vi "TCP IP Command Tester.vi"() -> ()   [LabVIEW 2015]
uses:
  Controls/Control_Fornax Set Monopolar Command - Coag Mode Enum.ctl
  Controls/Control_Fornax Set Monopolar Command - Serial Number String.ctl
  Controls/Control_Fornax Set Monopolar Command - Energy Channel ID Enum.ctl
  Controls/Control_Fornax Set Monopolar Command - Cut Mode Enum.ctl
  Controls/Control_Fornax Set Monopolar Command - Cut Power Command Enum.ctl
  Controls/Control_Fornax Set Monopolar Command - Coag Power Command Enum.ctl
  Controls/Control_Fornax Source ID.ctl
  Controls/Control_Fornax Switch ID.ctl
  Controls/Control_Fornax Energy Channel ID.ctl
  Controls/Control_Fornax Switch State.ctl
  Controls/Control_Fornax Energy Mode.ctl
  Controls/Control_Fornax Parameter Value.ctl
  Controls/Control_Fornax Parameter Type.ctl
  Controls/Control_Fornax Instrument Type.ctl
  Controls/Control_Fornax Mono1 Cut Increase Power.ctl
  Controls/Control_Fornax Mono1 Cut Decrease Power.ctl
  Controls/Control_Fornax Mono1 Coag Increase Power.ctl
  Controls/Control_Fornax Mono1 Coag Decrease Power.ctl
  Controls/Control_Fornax Mono1 Cut Enum.ctl
  Controls/Control_Fornax Mono1 Coag Enum.ctl
  Controls/Control_Fornax Mono1 Cut Activate Port Bool.ctl
  Controls/Control_Fornax Mono1 Coag Activate Port Bool.ctl
  Controls/Control_Fornax Mono2 Cut Activate Port Bool.ctl
  Controls/Control_Fornax Mono2 Coag Activate Port Bool.ctl
  Controls/Control_Fornax Mono2 Cut Decrease Power.ctl
  Controls/Control_Fornax Mono2 Cut Increase Power.ctl
  Controls/Control_Fornax Mono2 Cut Enum.ctl
  Controls/Control_Fornax Mono2 Coag Decrease Power.ctl
  Controls/Control_Fornax Mono2 Coag Increase Power.ctl
  Controls/Control_Fornax Mono2 Coag Enum.ctl
  Controls/Control_Fornax Bipolar Increase Power.ctl
  Controls/Control_Fornax Bipolar Decrease Power.ctl
  Controls/Control_Fornax Bipolar Enum.ctl
  Controls/Control_Fornax Bipolar Activate Port Bool.ctl
  Controls/Control_Fornax Ligasure Activate Port Bool.ctl
  Controls/QMH Fundamentals - Message Cluster.ctl
  Controls/Control_Fornax Generator.ctl
panel:
  in  "Stop":bool
  in  "Tab Control":T1(tab)
  in  "error in (no error)":errorcluster
  out "output cluster":T2
  out "Array":T3(array[cluster])
  in  "Fornax Executable Path":path=path "C:/Program Files (x86)/Medtronic/Fornax/x86/Fornax.exe"
  in  "Action 1":bool
  in  "ExternalCommCommand":T4(ring)=enum."EXTERNAL_COMM_COMMAND_PAIR_INTEGRATION_TESTOR"
  out "Display Message":string="Wait while TCP Connection established"
  in  "Set Monopolar Command":bool
  in  "CoagMode":T5
  in  "Serial Number":T6="T5G00443DX"
  in  "EnergyChannelID":T7
  in  "CutMode":T8
  in  "CutPowerCommand":T9
  in  "CoagPowerCommand":T10
  in  "Other Read Command":bool
  out "Display Message page 2":string="Wait while TCP Connection established"
  in  "String Command":string
  in  "Send String Command":bool
  out "String":string
  in  "Numeric (0-8)":i32
  in  "Send String Array Command":bool
  out "status":bool
  out "status 2":bool
  out "value read 2":string
  in  "Slider Status Command":bool
  in  "Switch Status Command":bool
  in  "System Config":bool
  in  "External Command":bool
  in  "External Command":T4(ring)
  in  "System Config":T11(ring)
  in  "Source ID":T12
  in  "Switch ID":T13
  in  "Switch State":T14
  in  "Energy Channel ID":T15
  in  "Energy Channel ID 2":T15
  in  "Slider Position":i32
  in  "Energy Parameter Command":bool
  in  "On/Off":bool
  in  "Mode":enum16{"Cut", "Coag", "Bipolar", "Ligasure"}(ring)
  in  "Port":enum16{"Mono1", "Mono2", "Bipolar", "Ligasure"}(ring)
  in  "Energy Mode":T16
  in  "Instrument Type":T17
  in  "Parameter Type":T18
  in  "Parameter Value":T19
  in  "Energy Channel ID 3":T15
  out "value read":string
  in  "timeout ms (25000)":i32
  in  "bytes to read":i32
  in  "mode (standard)":T20(ring)
  in  "Send Read Command":bool
  out "Mono1 - Bipolar Power":string
  out "Mono2 - Cut Power":string
  out "Mono1 - Coag Power":string
  out "Mono1 - Cut Power":string
  in  "Ligasure Activate":T21
  in  "Bipolar Activate":T22
  in  "Bipolar Enum":T23
  in  "Bipolar minus":T24
  in  "Bipolar plus":T25
  in  "Mono2 Coag Enum":T26=enum."Spray"
  in  "Mono2 Coag plus":T27
  in  "Mono2 Coag minus":T28
  in  "Mono2 Cut Enum":T29
  in  "Mono2 Cut plus":T30
  in  "Mono2 Cut minus":T31
  in  "Mono2 Coag Activate":T32
  in  "Mono2 Cut Activate":T33
  in  "Mono1 Coag Activate":T34
  in  "Mono1 Cut Activate":T35
  in  "Mono1 Coag Enum":T36=enum."Spray"
  in  "Mono1 Cut Enum":T37
  in  "Mono1 Coag minus":T38
  in  "Mono1 Coag plus":T39
  in  "Mono1 Cut minus":T40
  in  "Mono1 Cut plus":T41
  out "Mono2 - Coag Power":string
  in  "Test Read":bool
  in  "Slow Read":bool
  out "value read 3":string
  out "Open Bracket Found":bool
  out "Open Bracket":string
  out "Close Bracket Found":bool
  out "Current Read":string
  in  "Timeout":dbl=5.0 format="%#_13g"
  in  "milliseconds to wait":u32=100
  out "JSON Message":string[](array[string])
  # "Mono1"
  # "Mono2"
  # "Bipolar"
  # "Ligasure"
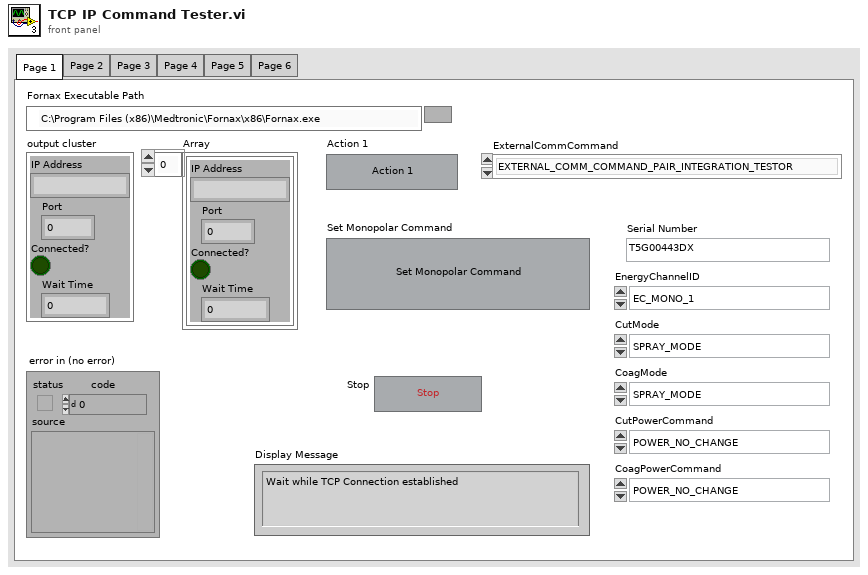
[diagram p1: front panel]
types:
  T1 = enum32{"Page 1", "Page 2", "Page 3", "Page 4", "Page 5", "Page 6"}
  T2 = cluster{"IP Address":string, "Port":u16, "Connected?":bool, "Wait Time":dbl}
  T3 = cluster{"IP Address":string, "Port":u16, "Connected?":bool, "Wait Time":dbl}[]
  T4 = enum16{"EXTERNAL_COMM_COMMAND_INVALID", "EXTERNAL_COMM_COMMAND_PAIR_VLEX", "EXTERNAL_COMM_COMMAND_PAIR_FORNAX", "EXTERNAL_COMM_COMMAND_PAIR_INTEGRATION_TESTOR", "EXTERNAL_COMM_COMMAND_ENABLE_DFA", "EXTERNAL_COMM_COMMAND_ENABLE_DFT", "EXTERNAL_COMM_COMMAND_ENABLE_VIPER", "EXTERNAL_COMM_COMMAND_AUTO_ETHERNET_ON", "EXTERNAL_COMM_COMMAND_AUTO_ETHERNET_OFF", "EXTERNAL_COMM_COMMAND_STREAM_RFDATA_ON", "EXTERNAL_COMM_COMMAND_STREAM_RFDATA_OFF", "EXTERNAL_COMM_COMMAND_STREAM_ISOFIRM_ON", "EXTERNAL_COMM_COMMAND_STREAM_ISOFIRM_OFF", "EXTERNAL_COMM_COMMAND_STREAM_RFID_ON", "EXTERNAL_COMM_COMMAND_STREAM_RFID_OFF", "EXTERNAL_COMM_COMMAND_AUTO_ETHERNET_ONCE"}
  T5 = typedef "Control_Fornax Set Monopolar Command - Coag Mode Enum.ctl" = enum16{"SPRAY_MODE", "CUT_MODE", "BLEND_MODE", "FULGERATE_MODE", "BEPOLAR_MODE", "VESSEL_SEALING_MODE", "VALLEYLAB_MODE", "BIPOLAR_RESECTION_CUT_MODE", "BIPOLAR_RESECTION_COAG_MODE", "AUTOBIPOLAR_MODE", "VIPER_HLA", "SOFT_COAG_MODE", "NUM_ENERGY_MODES"}
  T6 = typedef "Control_Fornax Set Monopolar Command - Serial Number String.ctl" = string
  T7 = typedef "Control_Fornax Set Monopolar Command - Energy Channel ID Enum.ctl" = enum16{"EC_MONO_1", "EC_BIPOLAR", "EC_MONO_2", "EC_ADVANCED", "NUM_ENERGY_CHANNELS", "EC_NOT_USED"}
  T8 = typedef "Control_Fornax Set Monopolar Command - Cut Mode Enum.ctl" = enum16{"SPRAY_MODE", "CUT_MODE", "BLEND_MODE", "FULGERATE_MODE", "BIPOLAR_MODE", "VESSEL_SEALING_MODE", "VALLEYLAB_MODE", "BIPOLAR_RESECTION_CUT_MODE", "BIPOLAR_RESECTION_COAG_MODE", "AUTOBIPOLAR_MODE", "VIPER_HLA", "SOFT_COAG_MODE", "NUM_ENERGY_MODES"}
  T9 = typedef "Control_Fornax Set Monopolar Command - Cut Power Command Enum.ctl" = enum16{"POWER_NO_CHANGE", "POWER_INCREASE", "POWER_DECREASE", "POWER_INCREASE_REPEAT", "POWER_DECREASE_REPEAT"}
  T10 = typedef "Control_Fornax Set Monopolar Command - Coag Power Command Enum.ctl" = enum16{"POWER_NO_CHANGE", "POWER_INCREASE", "POWER_DECREASE", "POWER_INCREASE_REPEAT", "POWER_DECREASE_REPEAT"}
  T11 = enum16{"SYSTEM_CONFIG_CMD_NONE", "SYSTEM_CONFIG_CMD_READ_CONFIG", "SYSTEM_CONFIG_CMD_WRITE_CONFIG", "SYSTEM_CONFIG_CMD_SW_UPDATE_ENTER", "SYSTEM_CONFIG_CMD_SW_UPDATE_START", "SYSTEM_CONFIG_CMD_SW_UPDATE_EXIT", "SYSTEM_CONFIG_CMD_UPDATE_ONE_BOARD_CHASSIS_INFO", "SYSTEM_CONFIG_CMD_UPDATE_ALL_BOARDS_CHASSIS_INFO", "SYSTEM_CONFIG_CMD_READ_ONE_BOARD_INFO", "SYSTEM_CONFIG_CMD_READ_ALL_BOARDS_INFO", "SYSTEM_CONFIG_CMD_REGISTER_BOARD", "SYSTEM_CONFIG_CMD_APPROVE_CURRENT_CONFIG", "SYSTEM_CONFIG_CMD_ROTATE_EVENT_LOGS", "SYSTEM_CONFIG_CMD_SYSTEM_RESTART", "SYSTEM_CONFIG_CMD_ROTATE_USAGE_LOGS", "SYSTEM_CONFIG_CMD_ENTER_SERVICE", "SYSTEM_CONFIG_CMD_EXIT_SERVICE", "SYSTEM_CONFIG_CMD_SW_UPDATE_CONFIRM", "SYSTEM_CONFIG_CMD_ROTATE_ALL_LOGS"}
  T12 = typedef "Control_Fornax Source ID.ctl" = enum16{"SWITCH_SOURCE_UNKNOWN  ", "SWITCH_SOURCE_HANDSWITCH  ", "SWITCH_SOURCE_FOOTSWITCH  ", "SWITCH_SOURCE_AUTO_BIPOLAR  ", "SWITCH_SOURCE_CARDIOBLATE  ", "SWITCH_SOURCE_SCREEN  ", "NUM_SWITCH_SOURCES  "}
  T13 = typedef "Control_Fornax Switch ID.ctl" = enum16{"SWITCH_ID_NONE  ", "SWITCH_ID_CUT  ", "SWITCH_ID_VMODE  ", "SWITCH_ID_COAG  ", "SWITCH_ID_LIGASURE  ", "SWITCH_ID_BIPOLAR  ", "SWITCH_ID_STAPLER_CLOSE  ", "SWITCH_ID_STAPLER_OPEN  ", "SWITCH_ID_CARDIOBLATE_BIPOLAR  ", "SWITCH_ID_CARDIOBLATE_BIPOLAR_TOUCHSCREEN  ", "SWITCH_ID_CARDIOBLATE_MONOPOLAR  ", "SWITCH_ID_CARDIOBLATE_MONOPOLAR_TOUCHSCREEN  ", "SWITCH_ID_ULTRASONIC_BTN1  ", "SWITCH_ID_ULTRASONIC_BTN2  ", "SWITCH_ID_MAX  "}
  T14 = typedef "Control_Fornax Switch State.ctl" = enum16{"SWITCH_STATE_NULL  ", "SWITCH_STATE_PRESSED  ", "SWITCH_STATE_RELEASED  ", "NUM_SWITCH_STATES  "}
  T15 = typedef "Control_Fornax Energy Channel ID.ctl" = enum16{"EC_MONO_1  ", "EC_BIPOLAR  ", "EC_MONO_2  ", "EC_ADVANCED  ", "EC_ADVANCED_ECUT  ", "EC_ADVANCED_DCUT  ", "EC_SHARED_COAG  ", "EC_INTERNAL_BIP_CAL  "}
  T16 = typedef "Control_Fornax Energy Mode.ctl" = enum16{"SPRAY_MODE", "CUT_MODE", "BLEND_MODE", "FULGERATE_MODE", "BIPOLAR_MODE", "VESSEL_SEALING_MODE", "VALLEYLAB_MODE", "BIPOLAR_RESECTION_CUT_MODE", "BIPOLAR_RESECTION_COAG_MODE", "AUTOBIPOLAR_MODE", "VIPER_HLA", "SOFT_COAG_MODE", "ECUT_MODE", "SHARED_SPRAY_MODE", "SHARED_FULGERATE_MODE", "CARDIO_MONO_MODE", "CARDIO_BIPOLAR_MODE", "BIPOLAR_LOW_MODE", "BIPOLAR_MACRO_MODE", "BIPOLAR_STANDARD_MODE", "BIPOLAR_MEDIUM_MODE", "VL_ENDOSCOPY_MODE", "NUM_ENERGY_MODES"}
  T17 = typedef "Control_Fornax Instrument Type.ctl" = enum16{"INSTRUMENT_TYPE_UNKNOWN", "INSTRUMENT_TYPE_MONOPOLAR", "INSTRUMENT_TYPE_BIPOLAR", "INSTRUMENT_TYPE_TRIVERSE", "INSTRUMENT_TYPE_LIGASURE", "INSTRUMENT_TYPE_ADVANCE_II", "INSTRUMENT_TYPE_BIPOLAR_RESECTION", "INSTRUMENT_TYPE_HOOK", "INSTRUMENT_TYPE_BIZACT", "INSTRUMENT_TYPE_CARDIOBLATE_BIP", "INSTRUMENT_TYPE_CARDIOBLATE_BIP_GEMINI_S", "INSTRUMENT_TYPE_CARDIOBLATE_MONO", "INSTRUMENT_TYPE_ULTRASONIC", "INSTRUMENT_TYPE_MONOPOLAR_GI ", "INSTRUMENT_TYPE_GOLDILOCKS "}
  T18 = typedef "Control_Fornax Parameter Type.ctl" = enum16{"POWER_PARAMETER", "CUT_MODALITY_POWER_PARAMETER", "COAG_MODALITY_POWER_PARAMETER", "VL_MODALITY_POWER_PARAMETER", "BY_MODE_POWER_PARAMETER", "VL_ENDO_CUT_MODALITY_POWER_PARAMETER", "VL_ENDO_COAG_MODALITY_POWER_PARAMETER", "VL_ENDO_COAG_ON_CUT_MODALITY_POWER_PARAMETER", "MODE_PARAMETER   (for changing Bipolar mode)", "CUT_MODALITY_MODE_PARAMETER  (for changing monopolar cut mode)", "COAG_MODALITY_MODE_PARAMETER (for changing monopolar coag mode)", "VL_ENDO_COAG_MODALITY_MODE_PARAMETER", "VL_ENDO_CUT_INTERVAL_PARAMETER", "VL_ENDO_CUT_DURATION_PARAMETER", "POWER_BAR_PARAMETER", "MAX_ACTIVATION_MSEC_TIME_PARAMETER", "AUTOBIPOLAR_DELAY_MSEC_TIME", "VL_ENDO_COAG_QUICK_ACCESS_PARAMETER"}
  T19 = typedef "Control_Fornax Parameter Value.ctl" = i32
  T20 = enum16{"Standard", "Buffered", "CRLF", "Immediate"}
  T21 = typedef "Control_Fornax Ligasure Activate Port Bool.ctl" = bool
  T22 = typedef "Control_Fornax Bipolar Activate Port Bool.ctl" = bool
  T23 = typedef "Control_Fornax Bipolar Enum.ctl" = enum16{"Standard", "Macro", "Precision"}
  T24 = typedef "Control_Fornax Bipolar Decrease Power.ctl" = bool
  T25 = typedef "Control_Fornax Bipolar Increase Power.ctl" = bool
  T26 = typedef "Control_Fornax Mono2 Coag Enum.ctl" = enum16{"Fulgerate", "Spray"}
  T27 = typedef "Control_Fornax Mono2 Coag Increase Power.ctl" = bool
  T28 = typedef "Control_Fornax Mono2 Coag Decrease Power.ctl" = bool
  T29 = typedef "Control_Fornax Mono2 Cut Enum.ctl" = enum16{"Pure", "Blend"}
  T30 = typedef "Control_Fornax Mono2 Cut Increase Power.ctl" = bool
  T31 = typedef "Control_Fornax Mono2 Cut Decrease Power.ctl" = bool
  T32 = typedef "Control_Fornax Mono2 Coag Activate Port Bool.ctl" = bool
  T33 = typedef "Control_Fornax Mono2 Cut Activate Port Bool.ctl" = bool
  T34 = typedef "Control_Fornax Mono1 Coag Activate Port Bool.ctl" = bool
  T35 = typedef "Control_Fornax Mono1 Cut Activate Port Bool.ctl" = bool
  T36 = typedef "Control_Fornax Mono1 Coag Enum.ctl" = enum16{"Fulgerate", "Spray"}
  T37 = typedef "Control_Fornax Mono1 Cut Enum.ctl" = enum16{"Pure", "Blend"}
  T38 = typedef "Control_Fornax Mono1 Coag Decrease Power.ctl" = bool
  T39 = typedef "Control_Fornax Mono1 Coag Increase Power.ctl" = bool
  T40 = typedef "Control_Fornax Mono1 Cut Decrease Power.ctl" = bool
  T41 = typedef "Control_Fornax Mono1 Cut Increase Power.ctl" = bool
  T42 = cluster{"Mono1 Cut Enum":refnum<vi>, "Mono1 - Cut Power":refnum<vi>, "Mono1 Coag Enum":refnum<vi>, "Mono1 - Coag Power":refnum<vi>, "Mono2 Cut Enum":refnum<vi>, "Mono2 - Cut Power":refnum<vi>, "Mono2 Coag Enum":refnum<vi>, "Mono2 - Coag Power":refnum<vi>, "Bipolar Enum":refnum<vi>, "Mono1 - Bipolar Power":refnum<vi>}
  T43 = typedef "QMH Fundamentals - Message Cluster.ctl" = cluster{"Message":string, "Message Data":variant}
  T44 = typedef "Control_Fornax Generator.ctl" = string
  T45 = cluster{"Port":enum16{"Mono1", "Mono2", "Bipolar", "Ligasure"}, "Mode":enum16{"Cut", "Coag", "Bipolar", "Ligasure"}, "On/Off":bool}
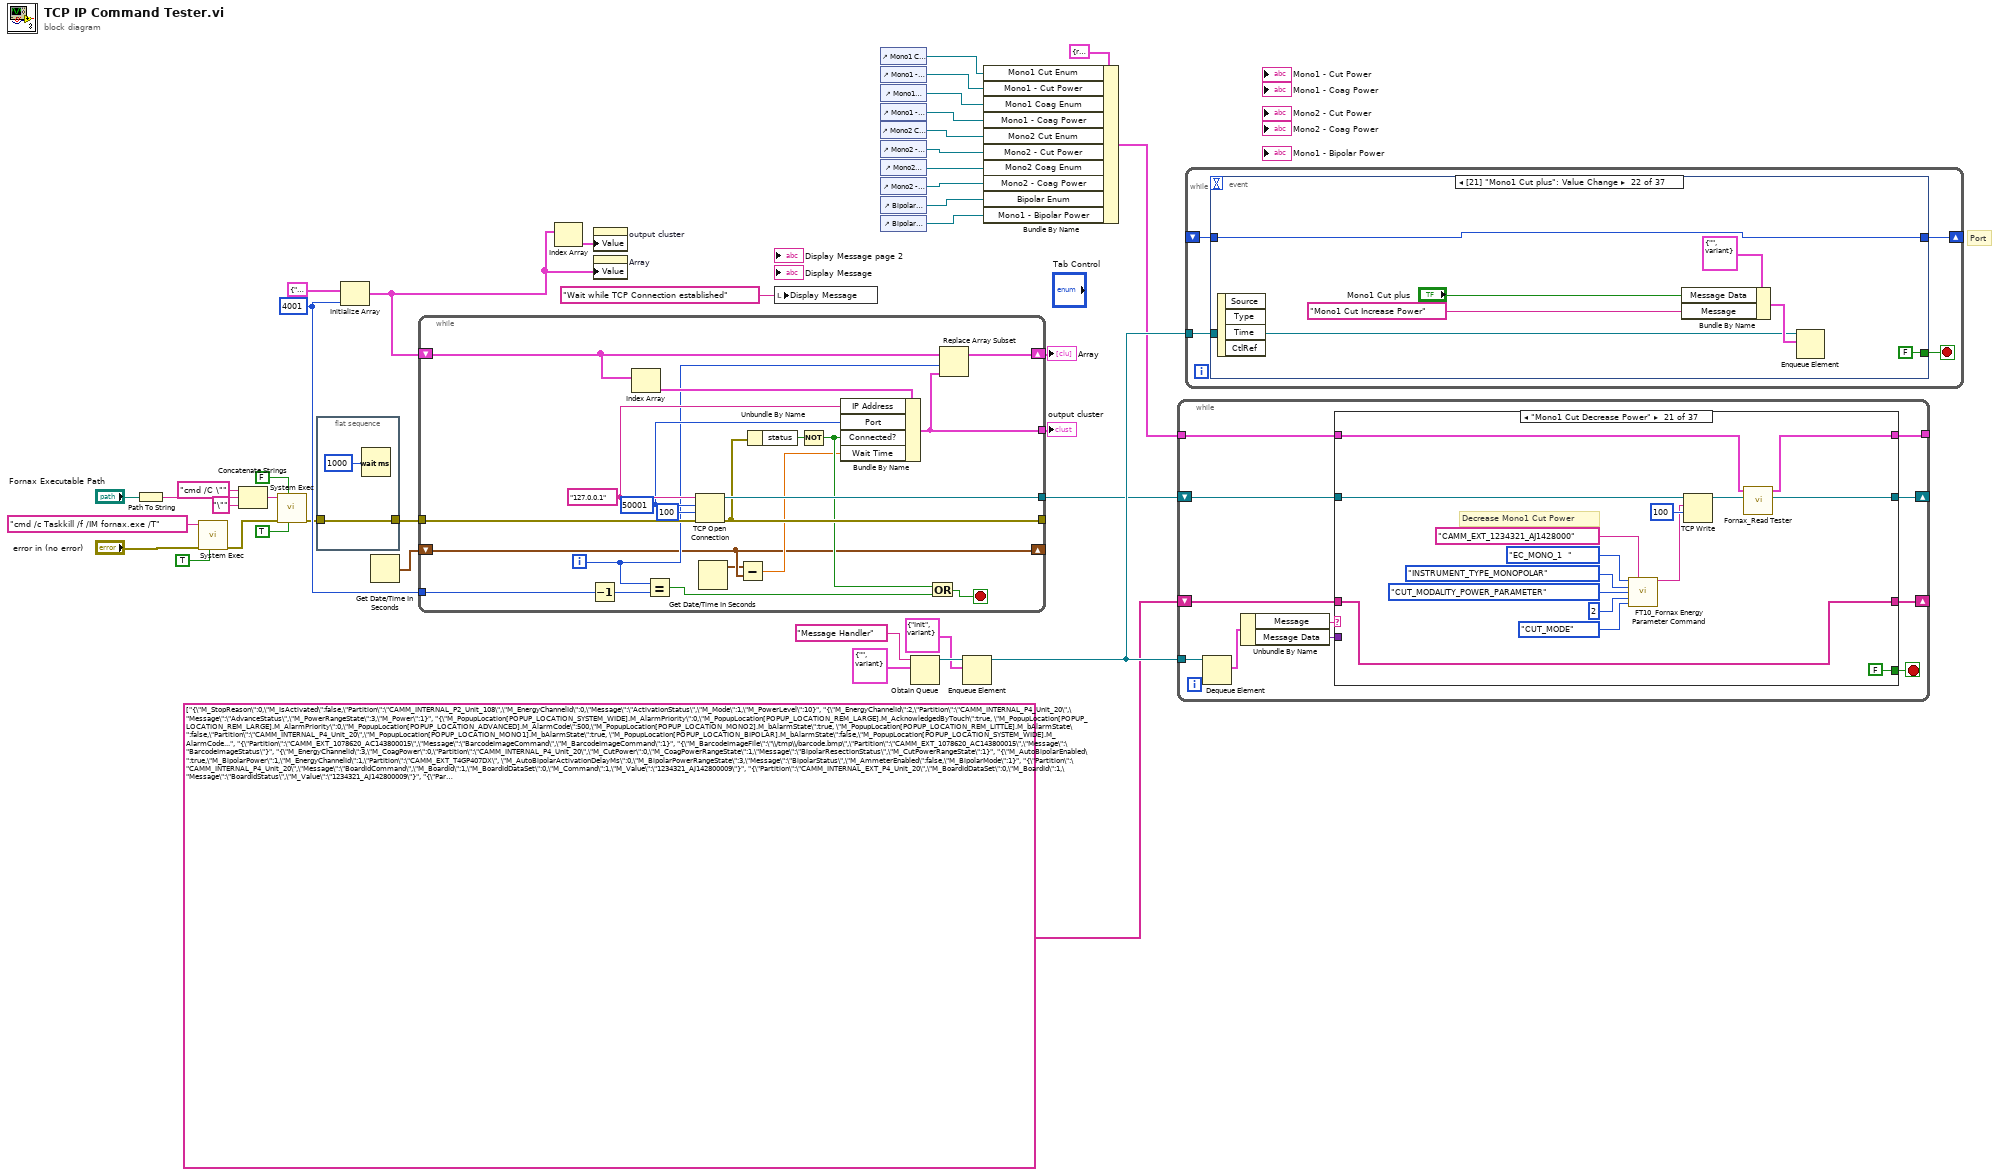
[diagram p0: block diagram]
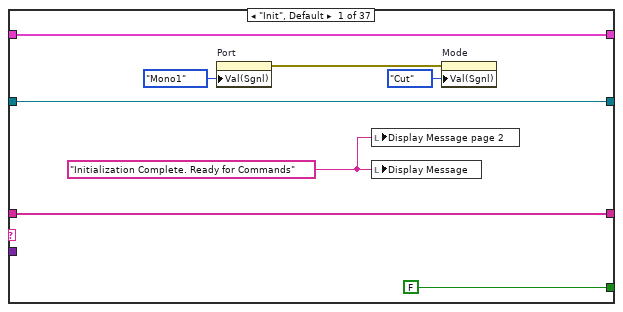
[diagram p2: hidden frame]
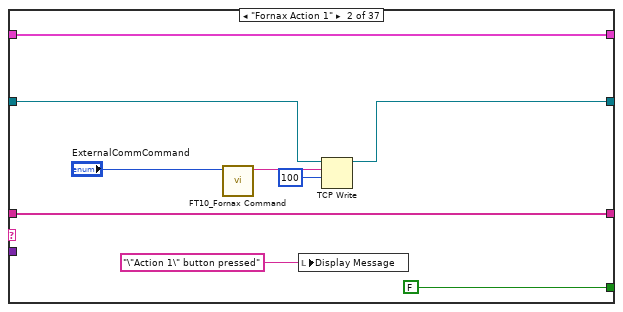
[diagram p3: hidden frame]
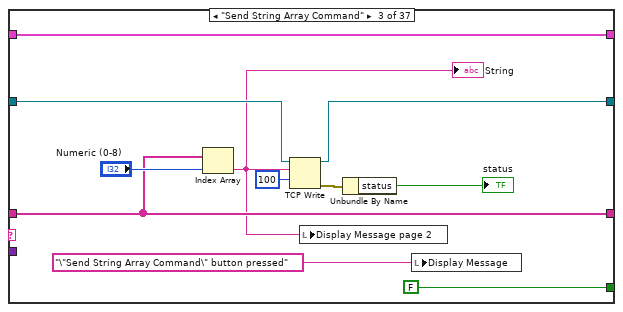
[diagram p4: hidden frame]
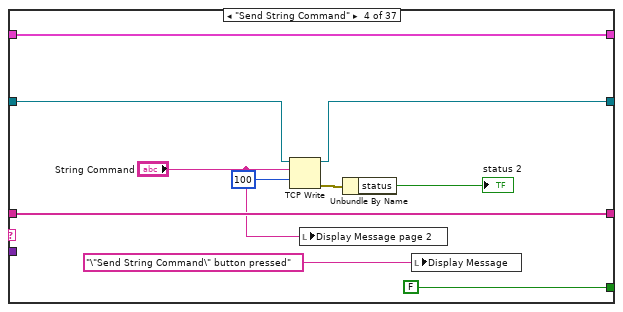
[diagram p5: hidden frame]
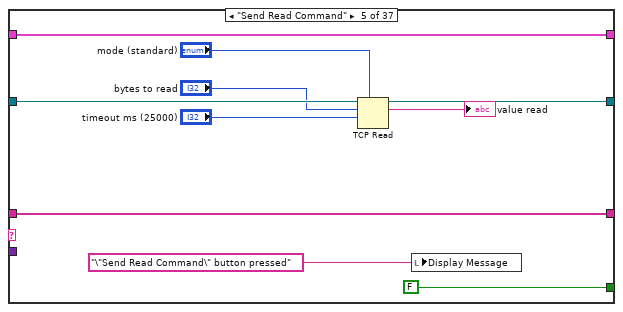
[diagram p6: hidden frame]
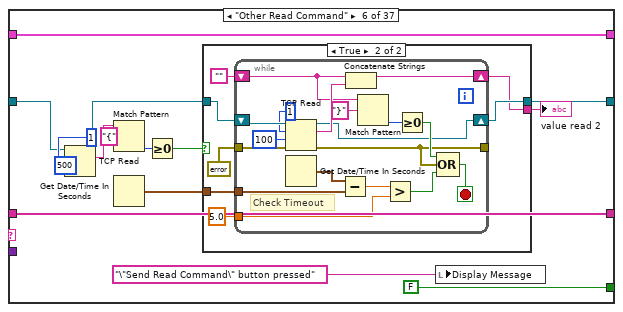
[diagram p7: hidden frame]
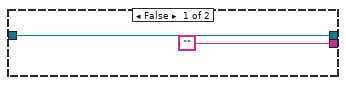
[diagram p8: hidden frame]
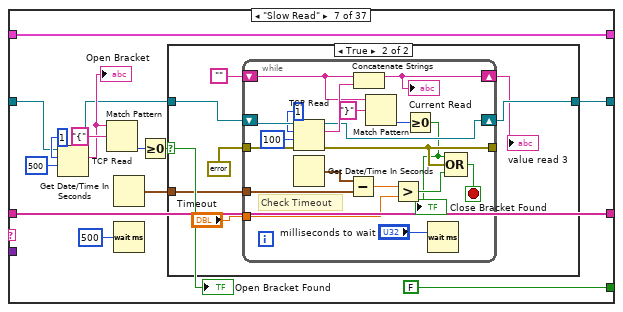
[diagram p9: hidden frame]
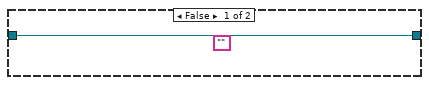
[diagram p10: hidden frame]
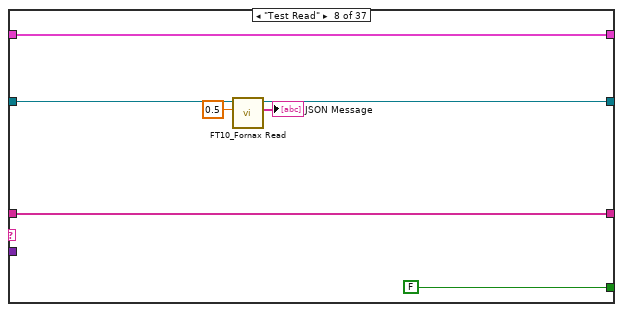
[diagram p11: hidden frame]
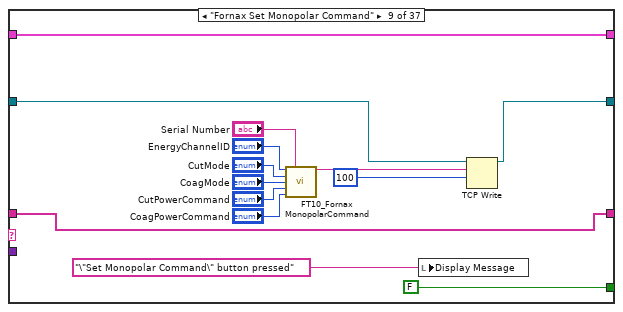
[diagram p12: hidden frame]
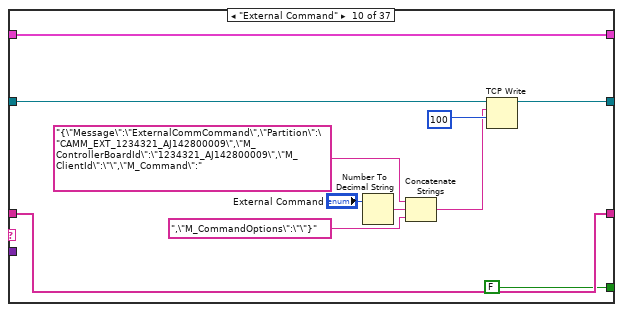
[diagram p13: hidden frame]
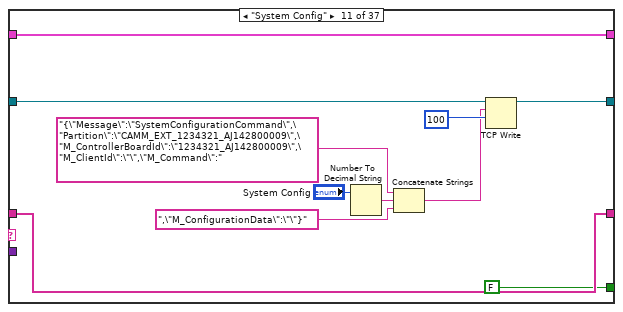
[diagram p14: hidden frame]
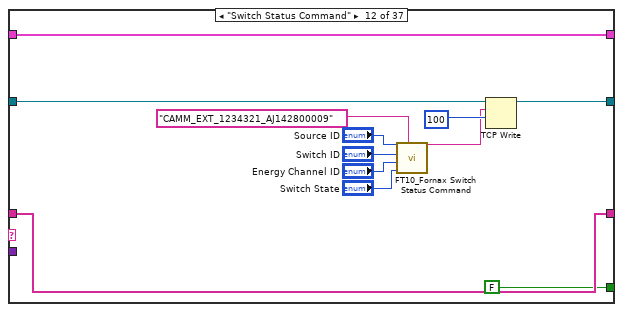
[diagram p15: hidden frame]
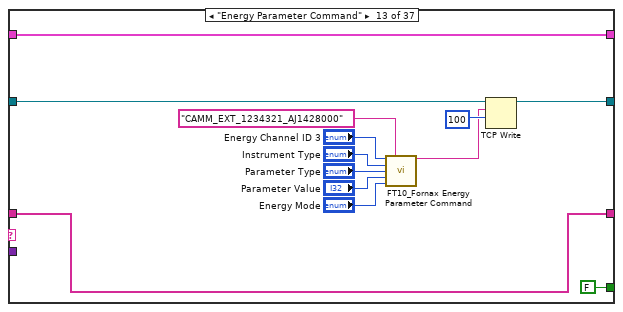
[diagram p16: hidden frame]
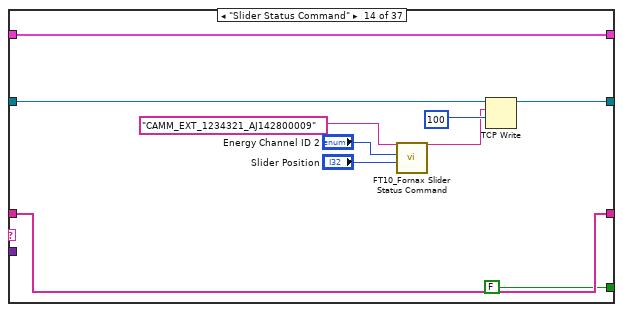
[diagram p17: hidden frame]
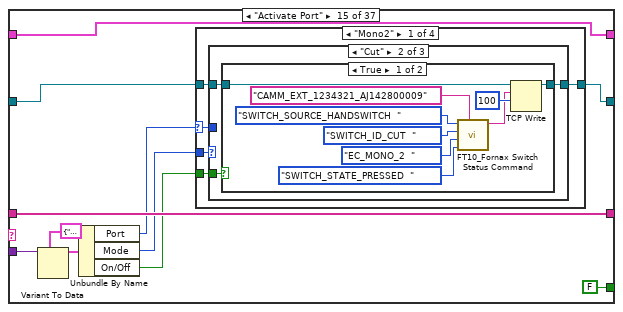
[diagram p18: hidden frame]
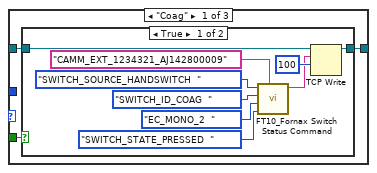
[diagram p19: hidden frame]
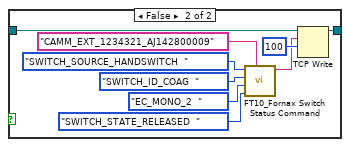
[diagram p20: hidden frame]
diagram:
  w38 = 4001 ("dimension size")
  # "Port"
  n1 = Path To String(path="Fornax Executable Path") -> (string=w27:string)
  n2 = call <vilib>:"System Exec.vi"("run minimized? (F)"=TRUE, "error in (no error)"="error in (no error)", "command line"="cmd /c Taskkill /f /IM fornax.exe /T") -> ("error out"=w33:errorcluster)  [unwired: 5 in, 3 out]
  n3 = Concatenate Strings("cmd /C \"" ("string"), w27, "\"" ("string")) -> (w29:string)
  n4 = call <vilib>:"System Exec.vi"("run minimized? (F)"=TRUE, "wait until completion? (T)"=FALSE, "error in (no error)"=w33, "command line"=w29) -> ("error out"=w13:errorcluster)  [unwired: 4 in, 3 out]
  n5 = flat-sequence {
    tunnel: [w42] -> w14
    tunnel: w13 -> [w42]
    frame #0 {
      n6 = Wait (ms)(milliseconds to wait=u32 1000) -> ()  [unwired: 1 out]
    }
  }
  n7 = Initialize Array(T2 {"IP Address"="", "Port"=0, "Connected?"=FALSE, "Wait Time"=0.0} ("Cluster"), w38) -> (w16:T3)
  n8 = Get Date/Time In Seconds() -> (seconds since 1Jan1904=w35:timestamp)
  n9 = while {
    tunnel: [w61] -> w19
    shift-right: [w60] -> w36
    shift-left: w16 -> [w59]
    tunnel: w38 -> [w50]
    tunnel: [w47] -> w37
    shift-right: [w44] -> _
    shift-left: w35 -> [w44]
    tunnel: w14 -> [w62]
    tunnel: [w55] -> _
    i -> [w46]
    stop <- w52 stop-if-true
    w56 = u16 50001 ("remote port or service name")
    w57 = "127.0.0.1" ("address")
    n10 = Decrement(x=w50) -> (x-1=w49:i32)
    n11 = Index Array(array=w59) -> (element=w58:T2)  [unwired: 1 in]
    n12 = Equal?(x=w46, y=w49) -> (x = y?=w48:bool)
    n13 = TCP Open Connection(address=w57, remote port or service name=w56, timeout ms (60000)=100, error in (no error)=w62) -> (connection ID=w61:refnum<k5>, error out=w55:errorcluster)  [unwired: 1 in]
    n14 = Get Date/Time In Seconds() -> (seconds since 1Jan1904=w43:timestamp)
    n15 = Subtract(x=w43, y=w44) -> (x-y=w45:dbl)
    n16 = Unbundle By Name(w55) -> ("status"=w54:bool)
    n17 = Not(x=w54) -> (.not. x?=w51:bool)
    n18 = Bundle By Name(cluster=w58, "IP Address"=w57, "Port"=w56, "Connected?"=w51, "Wait Time"=w45) -> (w47:T2)
    n19 = Or(x=w51, y=w48) -> (x .or. y?=w52:bool)
    n20 = Replace Array Subset(array=w59, new element=w47, index=w46) -> (w60:T3)
  }
  "output cluster" <- w37
  "Array" <- w36
  n21 = Index Array(array=w16) -> (element=w17:T2)  [unwired: 1 in]
  n22 = property on="output cluster" class="Clust (strict)"("Value"=w17) -> ()  [unwired: 2 in, 2 out]
  n23 = property on="Array" class="Arr (strict)"("Value"=w16) -> ()  [unwired: 2 in, 2 out]
  n24 = local write "Display Message"("Wait while TCP Connection established" ("Display Message")) -> ()
  n25 = control-ref of="Mono1 Cut Enum"() -> (w12:refnum<vi>)
  n26 = control-ref of="Mono1 - Cut Power"() -> (w5:refnum<vi>)
  n27 = control-ref of="Mono1 Coag Enum"() -> (w9:refnum<vi>)
  n28 = control-ref of="Mono1 - Coag Power"() -> (w4:refnum<vi>)
  n29 = control-ref of="Mono2 Cut Enum"() -> (w8:refnum<vi>)
  n30 = control-ref of="Mono2 - Cut Power"() -> (w3:refnum<vi>)
  n31 = control-ref of="Mono2 Coag Enum"() -> (w7:refnum<vi>)
  n32 = control-ref of="Mono2 - Coag Power"() -> (w2:refnum<vi>)
  n33 = control-ref of="Bipolar Enum"() -> (w6:refnum<vi>)
  n34 = control-ref of="Bipolar Power"() -> (w1:refnum<vi>)
  n35 = Obtain Queue(name (unnamed)="Message Handler", element data type=T43 {"Message"="", "Message Data"=variant} ("Message Cluster")) -> (queue out=w23:refnum<queue>)  [unwired: 3 in, 2 out]
  n36 = Enqueue Element(queue=w23, element=T43 {"Message"="Init", "Message Data"=variant}) -> (queue out=w20:refnum<queue>)  [unwired: 2 in, 2 out]
  n37 = Bundle By Name(cluster=T42 {"Mono1 Cut Enum"=refnum, "Mono1 - Cut Power"=refnum, "Mono1 Coag Enum"=refnum, "Mono1 - Coag Power"=refnum, "Mono2 Cut Enum"=refnum, "Mono2 - Cut Power"=refnum, "Mono2 Coag Enum"=refnum, "Mono2 - Coag Power"=refnum, "Bipolar Enum"=refnum, "Mono1 - Bipolar Power"=refnum}, "Mono1 Cut Enum"=w12, "Mono1 - Cut Power"=w5, "Mono1 Coag Enum"=w9, "Mono1 - Coag Power"=w4, "Mono2 Cut Enum"=w8, "Mono2 - Cut Power"=w3, "Mono2 Coag Enum"=w7, "Mono2 - Coag Power"=w2, "Bipolar Enum"=w6, "Mono1 - Bipolar Power"=w1) -> (w11:T42)
  n38 = while {
    tunnel: w20 -> [w72]
    shift-right: [w69] -> _
    shift-left: w19 -> [w68]
    shift-right: [w66] -> _
    shift-left: string[] ["{\"M_StopReason\":0,\"M_IsActivated\":false,\"Partition\":\"CAMM_INTERNAL_P2_Unit_108\",\"M_EnergyChannelId\":0,\"Message\":\"ActivationStatus\",\"M_Mode\":1,\"M_PowerLevel\":10}", "{\"M_EnergyChannelId\":2,\"Partition\":\"CAMM_INTERNAL_P4_Unit_20\",\"Message\":\"AdvanceStatus\",\"M_PowerRangeState\":3,\"M_Power\":1}", "{\"M_PopupLocation[POPUP_LOCATION_SYSTEM_WIDE].M_AlarmPriority\":0,\"M_PopupLocation[POPUP_LOCATION_REM_LARGE].M_AcknowledgedByTouch\":true, \"M_PopupLocation[POPUP_LOCATION_REM_LARGE].M_AlarmPriority\":0,\"M_PopupLocation[POPUP_LOCATION_ADVANCED].M_AlarmCode\":500,\"M_PopupLocation[POPUP_LOCATION_MONO2].M_bAlarmState\":true, \"M_PopupLocation[POPUP_LOCATION_REM_LITTLE].M_bAlarmState\":false,\"Partition\":\"CAMM_INTERNAL_P4_Unit_20\",\"M_PopupLocation[POPUP_LOCATION_MONO1].M_bAlarmState\":true, \"M_PopupLocation[POPUP_LOCATION_BIPOLAR].M_bAlarmState\":false,\"M_PopupLocation[POPUP_LOCATION_SYSTEM_WIDE].M_AlarmCode\":500,\"M_PopupLocation[POPUP_LOCATION_DEMO_MODE].M_AlarmCode\":500, \"M_PopupLocation[POPUP_LOCATION_SYSTEM_WIDE].M_AcknowledgedByTouch\":true,\"M_PopupLocation[POPUP_LOCATION_ADVANCED].M_AcknowledgedByTouch\":true, \"M_PopupLocation[POPUP_LOCATION_REM_LARGE].M_bAlarmState\":false,\"M_PopupLocation[POPUP_LOCATION_REM_LITTLE].M_AcknowledgedByTouch\":false,\"M_PopupLocation[POPUP_LOCATION_BIPOLAR].M_AlarmCode\":500, \"M_PopupLocation[POPUP_LOCATION_MONO1].M_AcknowledgedByTouch\":true,\"M_PopupLocation[POPUP_LOCATION_MONO1].M_AlarmCode\":331,\"M_PopupLocation[POPUP_LOCATION_REM_LITTLE].M_AlarmPriority\":0, \"Message\":\"AlarmPopupStatus\",\"M_PopupLocation[POPUP_LOCATION_DEMO_MODE].M_AcknowledgedByTouch\":true,\"M_PopupLocation[POPUP_LOCATION_MONO2].M_AlarmCode\":331, \"M_PopupLocation[POPUP_LOCATION_ADVANCED].M_AlarmPriority\":0,\"M_PopupLocation[POPUP_LOCATION_REM_LITTLE].M_AlarmCode\":500,\"M_PopupLocation[POPUP_LOCATION_BIPOLAR].M_AcknowledgedByTouch\":true, \"M_PopupLocation[POPUP_LOCATION_MONO1].M_AlarmPriority\":3,\"M_PopupLocation[POPUP_LOCATION_REM_LARGE].M_AlarmCode\":500,\"M_PopupLocation[POPUP_LOCATION_DEMO_MODE].M_bAlarmState\":false, \"M_PopupLocation[POPUP_LOCATION_SYSTEM_WIDE].M_bAlarmState\":false,\"M_PopupLocation[POPUP_LOCATION_MONO2].M_AcknowledgedByTouch\":true, \"M_PopupLocation[POPUP_LOCATION_BIPOLAR].M_AlarmPriority\":0,\"M_PopupLocation[POPUP_LOCATION_ADVANCED].M_bAlarmState\":false, \"M_PopupLocation[POPUP_LOCATION_DEMO_MODE].M_AlarmPriority\":0,\"M_PopupLocation[POPUP_LOCATION_MONO2].M_AlarmPriority\":3}", "{\"Partition\":\"CAMM_EXT_1078620_AC143800015\",\"Message\":\"BarcodeImageCommand\",\"M_BarcodeImageCommand\":1}", "{\"M_BarcodeImageFile\":\"\\/tmp\\/barcode.bmp\",\"Partition\":\"CAMM_EXT_1078620_AC143800015\",\"Message\":\"BarcodeImageStatus\"}", "{\"M_EnergyChannelId\":3,\"M_CoagPower\":0,\"Partition\":\"CAMM_INTERNAL_P4_Unit_20\",\"M_CutPower\":0,\"M_CoagPowerRangeState\":1,\"Message\":\"BipolarResectionStatus\",\"M_CutPowerRangeState\":1}", "{\"M_AutoBipolarEnabled\":true,\"M_BipolarPower\":1,\"M_EnergyChannelId\":1,\"Partition\":\"CAMM_EXT_T4GP407DX\", \"M_AutoBipolarActivationDelayMs\":0,\"M_BipolarPowerRangeState\":3,\"Message\":\"BipolarStatus\",\"M_AmmeterEnabled\":false,\"M_BipolarMode\":1}", "{\"Partition\":\"CAMM_INTERNAL_P4_Unit_20\",\"Message\":\"BoardIdCommand\",\"M_BoardId\":1,\"M_BoardIdDataSet\":0,\"M_Command\":1,\"M_Value\":\"1234321_AJ142800009\"}", "{\"Partition\":\"CAMM_INTERNAL_EXT_P4_Unit_20\",\"M_BoardIdDataSet\":0,\"M_BoardId\":1,\"Message\":\"BoardIdStatus\",\"M_Value\":\"1234321_AJ142800009\"}", "{\"Partition\":\"CAMM_INTERNAL_EXT_P4_Unit_20\",\"Message\":\"CardioblateBipolarStatus\",\"M_EnergyChannelId\":3,\"M_MaximumAblationTimeMS\":5,\"M_MaximumPowerLevel\":5}", "{\"Partition\":\"CAMM_INTERNAL_EXT_P4_Unit_20\",\"Message\":\"CardioblateMonopolarStatus\",\"M_CardioblateMonopolarPower\":5, \"M_CardioblateMonopolarPowerRangeState\":3,\"M_MaximumActivationTimeMS\":10,\"M_MaximumActivationTimeMSRangeState\":3}", "{\"Partition\":\"CAMM_INTERNAL_EXT_P4_Unit_20\",\"Message\":\"CardioblateSelectStatus\",\"M_SelectedEnergyChannel\":3}", "{\"Partition\":\"CAMM_EXT_1078620_AC143800015\",\"Message\":\"DftAlarmCommand\",\"M_ModuleId\":21,\"M_AlarmCode\":331, \"M_Command\":4,\"M_EnergyChannelId\":0,\"M_Message\":\"HELP\", \"M_CommandParams\":\"\",\"M_CommandOptions\":\"\"}", "{\"Partition\":\"CAMM_INTERNAL_EXT_P4_Unit_20\",\"M_AudioSequence\":1,\"Message\":\"DftAudioPlayCommand\",\"M_PlayMode\":3,\"M_Priority\":0,\"M_Volume\":50,\"M_OverrideSeqVolume\":false}", "{\"M_EnergyChannelId\":3,\"Partition\":\"CAMM_INTERNAL_EXT_P4_Unit_20\",\"Message\":\"DftInstrumentCommand\",\"M_DftInstrumentCommand\":1,\"M_IntValue\":0,\"M_FloatValue\":0.0,\"M_StringValue\":\"\"}", "{\"Partition\":\"CAMM_EXT_1078620_AC143800015\",\"Message\":\"DftLogCommand\",\"M_Command\":3,\"M_CommandOptions\":\"\"}", "{\"M_Command\":1,\"M_CalibrationType\":0,\"M_CalibrationTime\":\"\",\"M_Options\":\"\",\"M_EmA2dCalData.M_BipLowCurrentSecondary.M_Offset\":0.0,\"M_EmA2dCalData.M_BipLowCurrentPrimary.M_Gain\":1.0, \"M_EmA2dCalData.M_BipLowVoltPrimary.M_Gain\":1.0,\"Partition\":\"CAMM_INTERNAL_EXT_P4_Unit_20\",\"M_EmA2dCalData.M_BipHighVoltSecondary.M_Offset\":0.0,\"M_EmA2dCalData.M_BipLowVoltSecondary.M_Gain\":1.0, \"M_EmA2dCalData.M_BipLowVoltPrimary.M_Offset\":0.0,\"M_EmA2dCalData.M_BipHighVoltPrimary.M_Gain\":1.0,\"M_EmA2dCalData.M_MonoLowVoltPrimary.M_Offset\":0.0, \"M_EmA2dCalData.M_MonoLowVoltSecondary.M_Offset\":0.0,\"M_EmA2dCalData.M_BipHighCurrentSecondary.M_Offset\":0.0,\"M_EmA2dCalData.M_MonoLowVoltSecondary.M_Gain\":1.0, \"M_EmA2dCalData.M_BipHighCurrentPrimary.M_Gain\":1.0,\"M_EmA2dCalData.M_BipHighVoltSecondary.M_Gain\":1.0,\"M_EmA2dCalData.M_MonoHighVoltSecondary.M_Offset\":0.0, \"M_EmA2dCalData.M_BipHighCurrentPrimary.M_Offset\":0.0,\"Message\":\"EmA2dCalDataCommand\",\"M_EmA2dCalData.M_BipLowCurrentSecondary.M_Gain\":1.0, \"M_EmA2dCalData.M_BipLowCurrentPrimary.M_Offset\":0.0,\"M_EmA2dCalData.M_MonoHighVoltPrimary.M_Gain\":1.0, \"M_EmA2dCalData.M_BipHighCurrentSecondary.M_Gain\":1.0,\"M_EmA2dCalData.M_MonoHighVoltSecondary.M_Gain\":1.0, \"M_EmA2dCalData.M_BipHighVoltPrimary.M_Offset\":0.0,\"M_EmA2dCalData.M_MonoLowVoltPrimary.M_Gain\":1.0, \"M_EmA2dCalData.M_MonoHighVoltPrimary.M_Offset\":0.0,\"M_EmA2dCalData.M_BipLowVoltSecondary.M_Offset\":0.0}", "{\"M_EmA2dCalData.M_BipLowCurrentSecondary.M_Offset\":0.0,\"M_EmA2dCalData.M_BipLowCurrentPrimary.M_Gain\":1.01491,\"M_EmA2dCalData.M_BipLowVoltPrimary.M_Gain\":1.03926, \"Partition\":\"CAMM_EXT_1078620_AC143800029\",\"M_EmA2dCalData.M_BipHighVoltSecondary.M_Offset\":0.0,\"M_EmA2dCalData.M_BipLowVoltPrimary.M_Offset\":0.0, \"M_EmA2dCalData.M_BipLowVoltSecondary.M_Gain\":1.02606,\"M_EmA2dCalData.M_BipHighVoltPrimary.M_Gain\":1.03662,\"M_EmA2dCalData.M_MonoLowVoltPrimary.M_Offset\":0.0, \"M_EmA2dCalData.M_MonoLowVoltSecondary.M_Offset\":0.0,\"M_EmA2dCalData.M_BipHighCurrentSecondary.M_Offset\":0.0,\"M_EmA2dCalData.M_MonoLowVoltSecondary.M_Gain\":1.05138, \"M_EmA2dCalData.M_BipHighCurrentPrimary.M_Gain\":1.01475,\"M_EmA2dCalData.M_BipHighVoltSecondary.M_Gain\":1.02351,\"M_EmA2dCalData.M_MonoHighVoltSecondary.M_Offset\":0.0, \"M_EmA2dCalData.M_BipHighCurrentPrimary.M_Offset\":0.0,\"Message\":\"EmA2dCalDataStatus\",\"M_EmA2dCalData.M_BipLowCurrentSecondary.M_Gain\":1.0347, \"M_EmA2dCalData.M_BipLowCurrentPrimary.M_Offset\":0.0,\"M_EmA2dCalData.M_MonoHighVoltPrimary.M_Gain\":1.07264,\"M_EmA2dCalData.M_MonoHighVoltSecondary.M_Gain\":1.05568, \"M_EmA2dCalData.M_BipHighCurrentSecondary.M_Gain\":1.03478,\"M_Options\":\"\",\"M_EmA2dCalData.M_BipHighVoltPrimary.M_Offset\":0.0, \"M_CalibrationTime\":\"2014-11-18T00:26:27Z\", \"M_EmA2dCalData.M_MonoLowVoltPrimary.M_Gain\":1.06396,\"M_EmA2dCalData.M_MonoHighVoltPrimary.M_Offset\":0.0, \"M_CalibrationType\":-1,\"M_EmA2dCalData.M_BipLowVoltSecondary.M_Offset\":0.0}", "{\"Message\":\"EnergyParameterCommand\",\"Partition\":\"CAMM_EXT_1078620_AC143800015\",\"M_EnergyChannelId\":0;,\"M_InstrumentType\":1;,\"M_ParameterType\":1,\"M_ParameterValue\":3,\"M_EnergyMode\":-1}", "{\"Message\":\"ExternalCommCommand\",\"Partition\":\"CAMM_EXT_1078620_AC143800015\",\"M_ControllerBoardId\":\"1078620_AC143800015\",\"M_ClientId\":\"\",\"M_Command\":5,\"M_CommandOptions\":\"\"}"] ("String") -> [w65]
    tunnel: w11 -> [w63]
    tunnel: [w64] -> _
    stop <- w67 stop-if-true
    n39 = Dequeue Element(queue=w72) -> (element=w73:T43)  [unwired: 2 in, 3 out]
    n40 = Unbundle By Name(w73) -> ("Message"=w71:string, "Message Data"=w70:variant)
    n41 = case shown="\"Mono1 Cut Decrease Power\"" w71 {
      tunnel: w70 -> [_ _ _ _ _ _ _ _ _ _ _ _ _ _ w289 w455 _ _ w495 w505 _ _ w545 w555 _ _ w595 w605 _ _ w645 w655 _ _ w695 w705 _]
      tunnel: [w81 w86 w100 w110 w117 w134 w176 w207 w223 w235 w246 w258 w271 w281 w292 w452 w458 w474 w488 w501 w508 w523 w538 w550 w558 w573 w588 w599 w608 w623 w638 w649 w658 w673 w688 w700 w708] -> w69
      tunnel: w68 -> [w81 w87 w101 w111 w121 w126 w169 w208 w224 w236 w247 w259 w272 w282 w293 w453 w463 w484 w496 w502 w519 w534 w546 w551 w569 w584 w596 w600 w619 w634 w646 w651 w669 w684 w696 w702 w708]
      tunnel: [FALSE FALSE FALSE FALSE FALSE FALSE FALSE FALSE FALSE FALSE FALSE FALSE FALSE FALSE FALSE FALSE FALSE FALSE FALSE FALSE FALSE FALSE FALSE FALSE FALSE FALSE FALSE FALSE FALSE FALSE FALSE FALSE FALSE FALSE FALSE FALSE TRUE] -> w67
      tunnel: [w79 w83 w96 w107 w118 w123 w167 w209 w213 w233 w244 w256 w269 w279 w291 w451 w461 w476 w492 w504 w518 w533 w544 w554 w568 w583 w594 w604 w618 w633 w644 w654 w668 w683 w694 w704 w707] -> w66
      tunnel: w65 -> [w79 w83 w96 w107 w118 w123 w167 w209 w213 w233 w244 w256 w269 w279 w291 w451 w461 w476 w492 w504 w518 w533 w544 w554 w568 w583 w594 w604 w618 w633 w644 w654 w668 w683 w694 w704 w707]
      tunnel: [w74 w82 w91 w102 w112 w132 w175 w210 w212 w226 w237 w248 w260 w273 w283 w448 w456 w471 w486 w498 w506 w521 w536 w548 w556 w571 w586 w598 w606 w621 w636 w648 w656 w671 w686 w698 w706] -> w64
      tunnel: w63 -> [w74 w82 w91 w102 w112 w132 w175 w210 w212 w226 w237 w248 w260 w273 w283 w448 w457 w472 w487 w498 w507 w522 w537 w548 w557 w572 w587 w598 w607 w622 w637 w648 w657 w672 w687 w698 w706]
      frame "Init", Default {
        w78 = "Initialization Complete. Ready for Commands" ("Display Message")
        n42 = property on="Port" class="Enum (strict)"("Val(Sgnl)"=enum16{"Mono1", "Mono2", "Bipolar", "Ligasure"}."Mono1" ("Value (Signaling)")) -> (error out=w75:errorcluster)  [unwired: 2 in, 1 out]
        n43 = local write "Display Message page 2"(w78) -> ()
        n44 = local write "Display Message"(w78) -> ()
        n45 = property on="Mode" class="Enum (strict)"(error in=w75, "Val(Sgnl)"=enum16{"Cut", "Coag", "Bipolar", "Ligasure"}."Cut" ("Value (Signaling)")) -> ()  [unwired: 1 in, 2 out]
      }
      frame "Fornax Action 1" {
        n46 = call "FT10_Fornax Command.vi"("ExternalCommCommand"="ExternalCommCommand") -> ("JSON Message"=w89:string)  [unwired: 10 in]
        n47 = local write "Display Message"("\"Action 1\" button pressed" ("Display Message")) -> ()
        n48 = TCP Write(connection ID=w87, data in=w89, 9:100 ("timeout ms (25000)")) -> (connection ID out=w86:refnum<k5>)  [unwired: 1 in, 2 out]
      }
      frame "Send String Array Command" {
        n49 = Index Array(array=w96, index="Numeric (0-8)") -> (element=w92:string)
        "String" <- w92
        n50 = TCP Write(connection ID=w101, data in=w92, 9:100 ("timeout ms (25000)")) -> (connection ID out=w100:refnum<k5>, error out=w94:errorcluster)  [unwired: 1 in, 1 out]
        n51 = local write "Display Message page 2"(w92) -> ()
        n52 = Unbundle By Name(w94) -> ("status"=→"status":bool)
        n53 = local write "Display Message"("\"Send String Array Command\" button pressed" ("Display Message")) -> ()
      }
      frame "Send String Command" {
        n54 = TCP Write(connection ID=w111, data in="String Command", 9:100 ("timeout ms (25000)")) -> (connection ID out=w110:refnum<k5>, error out=w105:errorcluster)  [unwired: 1 in, 1 out]
        n55 = local write "Display Message page 2"("String Command") -> ()
        n56 = Unbundle By Name(w105) -> ("status"=→"status 2":bool)
        n57 = local write "Display Message"("\"Send String Command\" button pressed" ("Display Message")) -> ()
      }
      frame "Send Read Command" {
        n58 = TCP Read(connection ID=w121, bytes to read="bytes to read", 7:"mode (standard)", 9:"timeout ms (25000)") -> (connection ID out=w117:refnum<k5>, data out=→"value read":string)  [unwired: 1 in, 1 out]
        n59 = local write "Display Message"("\"Send Read Command\" button pressed" ("Display Message")) -> ()
      }
      frame "Other Read Command" {
        n60 = TCP Read(connection ID=w126, bytes to read=1, 9:500) -> (connection ID out=w125:refnum<k5>, data out=w127:string)  [unwired: 2 in, 1 out]
        n61 = Match Pattern(string=w127, regular expression="{") -> (offset past match=w128:i32)  [unwired: 1 in, 3 out]
        n62 = Get Date/Time In Seconds() -> (seconds since 1Jan1904=w122:timestamp)
        n63 = Greater Or Equal To 0?(x=w128) -> (x >= 0?=w124:bool)
        n64 = case shown="True" w124 {
          tunnel: [w138 w144] -> w134
          tunnel: ["" w143] -> w133
          tunnel: w125 -> [w138 w145]
          tunnel: w122 -> [_ w139]
          frame False {
          }
          frame True {
            n65 = while {
              tunnel: errorcluster {"status"=FALSE, "code"=0, "source"=""} ("error out") -> [w163]
              tunnel: [w149] -> _
              tunnel: w139 -> [w152]
              tunnel: 5.0 ("Timeout") -> [w159]
              shift-right: [w155] -> w143
              shift-left: "" -> [w148]
              shift-right: [w146] -> w144
              shift-left: w145 -> [w162]
              stop <- w157 stop-if-true
              # "Check Timeout"
              n66 = TCP Read(connection ID=w162, bytes to read=1, error in (no error)=w163, 9:100 ("timeout ms (25000)")) -> (connection ID out=w146:refnum<k5>, data out=w156:string, error out=w149:errorcluster)  [unwired: 1 in]
              n67 = Get Date/Time In Seconds() -> (seconds since 1Jan1904=w151:timestamp)
              n68 = Subtract(x=w151, y=w152) -> (x-y=w160:dbl)
              n69 = Concatenate Strings(w148, w156) -> (w155:string)
              n70 = Match Pattern(string=w148, regular expression="}") -> (offset past match=w161:i32)  [unwired: 1 in, 3 out]
              n71 = Greater?(x=w160, y=w159) -> (0:w158:bool)
              n72 = Greater Or Equal To 0?(x=w161) -> (x >= 0?=w150:bool)
              n73 = Compound Arithmetic op=OR(w150, w149, w158) -> (w157:bool)
            }
          }
        }
        "value read 2" <- w133
        n74 = local write "Display Message"("\"Send Read Command\" button pressed" ("Display Message")) -> ()
      }
      frame "Slow Read" {
        n75 = TCP Read(connection ID=w169, bytes to read=1, 9:500) -> (connection ID out=w168:refnum<k5>, data out=w170:string)  [unwired: 2 in, 1 out]
        "Open Bracket" <- w170
        n76 = Match Pattern(string=w170, regular expression="{") -> (offset past match=w171:i32)  [unwired: 1 in, 3 out]
        n77 = Get Date/Time In Seconds() -> (seconds since 1Jan1904=w166:timestamp)
        n78 = Wait (ms)(milliseconds to wait=u32 500) -> ()  [unwired: 1 out]
        n79 = Greater Or Equal To 0?(x=w171) -> (x >= 0?=w164:bool)
        "Open Bracket Found" <- w164
        n80 = case shown="True" w164 {
          tunnel: [w178 w184] -> w176
          tunnel: w168 -> [w178 w185]
          tunnel: w166 -> [_ w181]
          frame False {
            (unwired) ""
          }
          frame True {
            n81 = while {
              tunnel: errorcluster {"status"=FALSE, "code"=0, "source"=""} ("error out") -> [w204]
              tunnel: [w192] -> _
              tunnel: w181 -> [w194]
              tunnel: "Timeout" -> [w200]
              shift-right: [w186] -> w180
              shift-left: "" -> [w191]
              shift-right: [w189] -> w184
              shift-left: w185 -> [w203]
              stop <- w198 stop-if-true
              # "Check Timeout"
              n82 = TCP Read(connection ID=w203, bytes to read=1, error in (no error)=w204, 9:100 ("timeout ms (25000)")) -> (connection ID out=w189:refnum<k5>, data out=w197:string, error out=w192:errorcluster)  [unwired: 1 in]
              n83 = Get Date/Time In Seconds() -> (seconds since 1Jan1904=w193:timestamp)
              n84 = Subtract(x=w193, y=w194) -> (x-y=w201:dbl)
              n85 = Concatenate Strings(w191, w197) -> (w186:string)
              "Current Read" <- w186
              n86 = Match Pattern(string=w191, regular expression="}") -> (offset past match=w202:i32)  [unwired: 1 in, 3 out]
              n87 = Greater?(x=w201, y=w200) -> (0:w199:bool)
              n88 = Greater Or Equal To 0?(x=w202) -> (x >= 0?=w187:bool)
              "Close Bracket Found" <- w187
              n89 = Wait (ms)(milliseconds to wait="milliseconds to wait") -> ()  [unwired: 1 out]
              n90 = Compound Arithmetic op=OR(w187, w192, w199) -> (w198:bool)
            }
            "value read 3" <- w180
          }
        }
      }
      frame "Test Read" {
        n91 = call "FT10_Fornax Read.vi"("Timeout"=0.5, "TCP Network Connection in"=w208) -> ("JSON Message"=→"JSON Message":string[], "TCP Network Connection out"=w207:refnum<k5>)  [unwired: 7 in, 1 out]
      }
      frame "Fornax Set Monopolar Command" {
        n92 = call "FT10_Fornax MonopolarCommand.vi"("EnergyChannelID"="EnergyChannelID", "Serial Number"="Serial Number", "CutMode"="CutMode", "CoagMode"="CoagMode", "CutPowerCommand"="CutPowerCommand", "CoagPowerCommand"="CoagPowerCommand") -> ("JSON Command"=w220:string)  [unwired: 9 in]
        n93 = local write "Display Message"("\"Set Monopolar Command\" button pressed" ("Display Message")) -> ()
        n94 = TCP Write(connection ID=w224, data in=w220, 9:100 ("timeout ms (25000)")) -> (connection ID out=w223:refnum<k5>)  [unwired: 1 in, 2 out]
      }
      frame "External Command" {
        n95 = Number To Decimal String(number="External Command") -> (decimal integer string=w231:string)  [unwired: 1 in]
        n96 = Concatenate Strings("{\"Message\":\"ExternalCommCommand\",\"Partition\":\"CAMM_EXT_1234321_AJ142800009\",\"M_ControllerBoardId\":\"1234321_AJ142800009\",\"M_ClientId\":\"\",\"M_Command\":", w231, ",\"M_CommandOptions\":\"\"}") -> (w228:string)
        n97 = TCP Write(connection ID=w236, data in=w228, 9:100 ("timeout ms (25000)")) -> (connection ID out=w235:refnum<k5>)  [unwired: 1 in, 2 out]
      }
      frame "System Config" {
        n98 = Number To Decimal String(number="System Config") -> (decimal integer string=w242:string)  [unwired: 1 in]
        n99 = Concatenate Strings("{\"Message\":\"SystemConfigurationCommand\",\"Partition\":\"CAMM_EXT_1234321_AJ142800009\",\"M_ControllerBoardId\":\"1234321_AJ142800009\",\"M_ClientId\":\"\",\"M_Command\":", w242, ",\"M_ConfigurationData\":\"\"}") -> (w239:string)
        n100 = TCP Write(connection ID=w247, data in=w239, 9:100 ("timeout ms (25000)")) -> (connection ID out=w246:refnum<k5>)  [unwired: 1 in, 2 out]
      }
      frame "Switch Status Command" {
        n101 = call "FT10_Fornax Switch Status Command.vi"("Generator"=T44 "CAMM_EXT_1234321_AJ142800009", "Switch State"="Switch State", "Energy Channel ID"="Energy Channel ID", "Switch ID"="Switch ID", "Source ID"="Source ID") -> ("JSON Command"=w249:string)  [unwired: 6 in]
        n102 = TCP Write(connection ID=w259, data in=w249, 9:100 ("timeout ms (25000)")) -> (connection ID out=w258:refnum<k5>)  [unwired: 1 in, 2 out]
      }
      frame "Energy Parameter Command" {
        n103 = call "FT10_Fornax Energy Parameter Command.vi"("Energy Channel ID"="Energy Channel ID 3", "Generator"=T44 "CAMM_EXT_1234321_AJ1428000", "Instrument Type"="Instrument Type", "Parameter Type"="Parameter Type", "Parameter Value"="Parameter Value", "Energy Mode"="Energy Mode") -> ("JSON Command"=w261:string)  [unwired: 9 in]
        n104 = TCP Write(connection ID=w272, data in=w261, 9:100 ("timeout ms (25000)")) -> (connection ID out=w271:refnum<k5>)  [unwired: 1 in, 2 out]
      }
      frame "Slider Status Command" {
        n105 = call "FT10_Fornax Slider Status Command.vi"("Slider Position"="Slider Position", "Energy Channel ID"="Energy Channel ID 2", "Generator"=T44 "CAMM_EXT_1234321_AJ142800009") -> ("JSON Command"=w277:string)  [unwired: 8 in]
        n106 = TCP Write(connection ID=w282, data in=w277, 9:100 ("timeout ms (25000)")) -> (connection ID out=w281:refnum<k5>)  [unwired: 1 in, 2 out]
      }
      frame "Activate Port" {
        n107 = Variant To Data(type=T45 {"Port"=enum."Bipolar", "Mode"=enum."Bipolar", "On/Off"=FALSE}, Variant=w289) -> (data=w287:T45)  [unwired: 1 in, 1 out]
        n108 = Unbundle By Name(w287) -> ("Port"=w286:enum16{"Mono1", "Mono2", "Bipolar", "Ligasure"}, "Mode"=w285:enum16{"Cut", "Coag", "Bipolar", "Ligasure"}, "On/Off"=w284:bool)
        n109 = case shown="\"Mono2\"" w286 {
          selector: w286 -> [w296 w345 w394 w422]
          tunnel: w293 -> [w298 w347 w396 w424]
          tunnel: [w297 w346 w395 w423] -> w292
          tunnel: w285 -> [w295 w344 w393 w421]
          tunnel: w284 -> [w294 w343 w392 w420]
          frame "Mono2" {
            n110 = case shown="\"Cut\"" w295 {
              tunnel: w298 -> [w301 w322 w342]
              tunnel: [w300 w321 w342] -> w297
              tunnel: w296 -> [_ _ _]
              tunnel: w294 -> [w299 w320 _]
              frame "Coag" {
                n111 = case shown="True" w299 {
                  tunnel: w301 -> [w310 w319]
                  tunnel: [w309 w318] -> w300
                  frame True {
                    n112 = call "FT10_Fornax Switch Status Command.vi"("Generator"=T44 "CAMM_EXT_1234321_AJ142800009", "Switch State"=Control_Fornax_Switch_State."SWITCH_STATE_PRESSED  ", "Energy Channel ID"=Control_Fornax_Energy_Channel_ID."EC_MONO_2  ", "Switch ID"=Control_Fornax_Switch_ID."SWITCH_ID_COAG  ", "Source ID"=Control_Fornax_Source_ID."SWITCH_SOURCE_HANDSWITCH  ") -> ("JSON Command"=w302:string)  [unwired: 6 in]
                    n113 = TCP Write(connection ID=w310, data in=w302, 9:100 ("timeout ms (25000)")) -> (connection ID out=w309:refnum<k5>)  [unwired: 1 in, 2 out]
                  }
                  frame False {
                    n114 = call "FT10_Fornax Switch Status Command.vi"("Generator"=T44 "CAMM_EXT_1234321_AJ142800009", "Switch State"=Control_Fornax_Switch_State."SWITCH_STATE_RELEASED  ", "Energy Channel ID"=Control_Fornax_Energy_Channel_ID."EC_MONO_2  ", "Switch ID"=Control_Fornax_Switch_ID."SWITCH_ID_COAG  ", "Source ID"=Control_Fornax_Source_ID."SWITCH_SOURCE_HANDSWITCH  ") -> ("JSON Command"=w311:string)  [unwired: 6 in]
                    n115 = TCP Write(connection ID=w319, data in=w311, 9:100 ("timeout ms (25000)")) -> (connection ID out=w318:refnum<k5>)  [unwired: 1 in, 2 out]
                  }
                }
              }
              frame "Cut" {
                n116 = case shown="True" w320 {
                  tunnel: w322 -> [w331 w340]
                  tunnel: [w330 w339] -> w321
                  frame True {
                    n117 = call "FT10_Fornax Switch Status Command.vi"("Generator"=T44 "CAMM_EXT_1234321_AJ142800009", "Switch State"=Control_Fornax_Switch_State."SWITCH_STATE_PRESSED  ", "Energy Channel ID"=Control_Fornax_Energy_Channel_ID."EC_MONO_2  ", "Switch ID"=Control_Fornax_Switch_ID."SWITCH_ID_CUT  ", "Source ID"=Control_Fornax_Source_ID."SWITCH_SOURCE_HANDSWITCH  ") -> ("JSON Command"=w323:string)  [unwired: 6 in]
                    n118 = TCP Write(connection ID=w331, data in=w323, 9:100 ("timeout ms (25000)")) -> (connection ID out=w330:refnum<k5>)  [unwired: 1 in, 2 out]
                  }
                  frame False {
                    n119 = call "FT10_Fornax Switch Status Command.vi"("Generator"=T44 "CAMM_EXT_1234321_AJ142800009", "Switch State"=Control_Fornax_Switch_State."SWITCH_STATE_RELEASED  ", "Energy Channel ID"=Control_Fornax_Energy_Channel_ID."EC_MONO_2  ", "Switch ID"=Control_Fornax_Switch_ID."SWITCH_ID_CUT  ", "Source ID"=Control_Fornax_Source_ID."SWITCH_SOURCE_HANDSWITCH  ") -> ("JSON Command"=w332:string)  [unwired: 6 in]
                    n120 = TCP Write(connection ID=w340, data in=w332, 9:100 ("timeout ms (25000)")) -> (connection ID out=w339:refnum<k5>)  [unwired: 1 in, 2 out]
                  }
                }
              }
              frame Default {
                n121 = One Button Dialog(message="This mode is not allowed for this port") -> ()  [unwired: 1 in, 1 out]
              }
            }
          }
          frame "Mono1" {
            n122 = case shown="\"Coag\"" w344 {
              tunnel: w347 -> [w350 w371 w391]
              tunnel: [w349 w370 w391] -> w346
              tunnel: w345 -> [_ _ _]
              tunnel: w343 -> [w348 w369 _]
              frame "Coag" {
                n123 = case shown="False" w348 {
                  tunnel: w350 -> [w359 w368]
                  tunnel: [w358 w367] -> w349
                  frame True {
                    n124 = call "FT10_Fornax Switch Status Command.vi"("Generator"=T44 "CAMM_EXT_1234321_AJ142800009", "Switch State"=Control_Fornax_Switch_State."SWITCH_STATE_PRESSED  ", "Energy Channel ID"=Control_Fornax_Energy_Channel_ID."EC_MONO_1  ", "Switch ID"=Control_Fornax_Switch_ID."SWITCH_ID_COAG  ", "Source ID"=Control_Fornax_Source_ID."SWITCH_SOURCE_HANDSWITCH  ") -> ("JSON Command"=w351:string)  [unwired: 6 in]
                    n125 = TCP Write(connection ID=w359, data in=w351, 9:100 ("timeout ms (25000)")) -> (connection ID out=w358:refnum<k5>)  [unwired: 1 in, 2 out]
                  }
                  frame False {
                    n126 = call "FT10_Fornax Switch Status Command.vi"("Generator"=T44 "CAMM_EXT_1234321_AJ142800009", "Switch State"=Control_Fornax_Switch_State."SWITCH_STATE_RELEASED  ", "Energy Channel ID"=Control_Fornax_Energy_Channel_ID."EC_MONO_1  ", "Switch ID"=Control_Fornax_Switch_ID."SWITCH_ID_COAG  ", "Source ID"=Control_Fornax_Source_ID."SWITCH_SOURCE_HANDSWITCH  ") -> ("JSON Command"=w360:string)  [unwired: 6 in]
                    n127 = TCP Write(connection ID=w368, data in=w360, 9:100 ("timeout ms (25000)")) -> (connection ID out=w367:refnum<k5>)  [unwired: 1 in, 2 out]
                  }
                }
              }
              frame "Cut" {
                n128 = case shown="True" w369 {
                  tunnel: w371 -> [w380 w389]
                  tunnel: [w379 w388] -> w370
                  frame True {
                    n129 = call "FT10_Fornax Switch Status Command.vi"("Generator"=T44 "CAMM_EXT_1234321_AJ142800009", "Switch State"=Control_Fornax_Switch_State."SWITCH_STATE_PRESSED  ", "Energy Channel ID"=Control_Fornax_Energy_Channel_ID."EC_MONO_1  ", "Switch ID"=Control_Fornax_Switch_ID."SWITCH_ID_CUT  ", "Source ID"=Control_Fornax_Source_ID."SWITCH_SOURCE_HANDSWITCH  ") -> ("JSON Command"=w372:string)  [unwired: 6 in]
                    n130 = TCP Write(connection ID=w380, data in=w372, 9:100 ("timeout ms (25000)")) -> (connection ID out=w379:refnum<k5>)  [unwired: 1 in, 2 out]
                  }
                  frame False {
                    n131 = call "FT10_Fornax Switch Status Command.vi"("Generator"=T44 "CAMM_EXT_1234321_AJ142800009", "Switch State"=Control_Fornax_Switch_State."SWITCH_STATE_RELEASED  ", "Energy Channel ID"=Control_Fornax_Energy_Channel_ID."EC_MONO_1  ", "Switch ID"=Control_Fornax_Switch_ID."SWITCH_ID_CUT  ", "Source ID"=Control_Fornax_Source_ID."SWITCH_SOURCE_HANDSWITCH  ") -> ("JSON Command"=w381:string)  [unwired: 6 in]
                    n132 = TCP Write(connection ID=w389, data in=w381, 9:100 ("timeout ms (25000)")) -> (connection ID out=w388:refnum<k5>)  [unwired: 1 in, 2 out]
                  }
                }
              }
              frame Default {
                n133 = One Button Dialog(message="This mode is not allowed for this port") -> ()  [unwired: 1 in, 1 out]
              }
            }
          }
          frame "Bipolar" {
            n134 = case shown="\"Bipolar\"" w393 {
              tunnel: w396 -> [w399 w419]
              tunnel: [w398 w419] -> w395
              tunnel: w394 -> [_ _]
              tunnel: w392 -> [w397 _]
              frame "Bipolar" {
                n135 = case shown="False" w397 {
                  tunnel: w399 -> [w408 w417]
                  tunnel: [w407 w416] -> w398
                  frame True {
                    n136 = call "FT10_Fornax Switch Status Command.vi"("Generator"=T44 "CAMM_EXT_1234321_AJ142800009", "Switch State"=Control_Fornax_Switch_State."SWITCH_STATE_PRESSED  ", "Energy Channel ID"=Control_Fornax_Energy_Channel_ID."EC_BIPOLAR  ", "Switch ID"=Control_Fornax_Switch_ID."SWITCH_ID_BIPOLAR  ", "Source ID"=Control_Fornax_Source_ID."SWITCH_SOURCE_HANDSWITCH  ") -> ("JSON Command"=w400:string)  [unwired: 6 in]
                    n137 = TCP Write(connection ID=w408, data in=w400, 9:100 ("timeout ms (25000)")) -> (connection ID out=w407:refnum<k5>)  [unwired: 1 in, 2 out]
                  }
                  frame False {
                    n138 = call "FT10_Fornax Switch Status Command.vi"("Generator"=T44 "CAMM_EXT_1234321_AJ142800009", "Switch State"=Control_Fornax_Switch_State."SWITCH_STATE_RELEASED  ", "Energy Channel ID"=Control_Fornax_Energy_Channel_ID."EC_BIPOLAR  ", "Switch ID"=Control_Fornax_Switch_ID."SWITCH_ID_BIPOLAR  ", "Source ID"=Control_Fornax_Source_ID."SWITCH_SOURCE_HANDSWITCH  ") -> ("JSON Command"=w409:string)  [unwired: 6 in]
                    n139 = TCP Write(connection ID=w417, data in=w409, 9:100 ("timeout ms (25000)")) -> (connection ID out=w416:refnum<k5>)  [unwired: 1 in, 2 out]
                  }
                }
              }
              frame Default {
                n140 = One Button Dialog(message="This mode is not allowed for this port") -> ()  [unwired: 1 in, 1 out]
              }
            }
          }
          frame "Ligasure" {
            n141 = case shown="\"Ligasure\"" w421 {
              tunnel: w424 -> [w427 w447]
              tunnel: [w426 w447] -> w423
              tunnel: w422 -> [_ _]
              tunnel: w420 -> [w425 _]
              frame "Ligasure" {
                n142 = case shown="True" w425 {
                  tunnel: w427 -> [w436 w445]
                  tunnel: [w435 w444] -> w426
                  frame True {
                    n143 = call "FT10_Fornax Switch Status Command.vi"("Generator"=T44 "CAMM_EXT_1234321_AJ142800009", "Switch State"=Control_Fornax_Switch_State."SWITCH_STATE_PRESSED  ", "Energy Channel ID"=Control_Fornax_Energy_Channel_ID."EC_ADVANCED  ", "Switch ID"=Control_Fornax_Switch_ID."SWITCH_ID_LIGASURE  ", "Source ID"=Control_Fornax_Source_ID."SWITCH_SOURCE_HANDSWITCH  ") -> ("JSON Command"=w428:string)  [unwired: 6 in]
                    n144 = TCP Write(connection ID=w436, data in=w428, 9:100 ("timeout ms (25000)")) -> (connection ID out=w435:refnum<k5>)  [unwired: 1 in, 2 out]
                  }
                  frame False {
                    n145 = call "FT10_Fornax Switch Status Command.vi"("Generator"=T44 "CAMM_EXT_1234321_AJ142800009", "Switch State"=Control_Fornax_Switch_State."SWITCH_STATE_RELEASED  ", "Energy Channel ID"=Control_Fornax_Energy_Channel_ID."EC_ADVANCED  ", "Switch ID"=Control_Fornax_Switch_ID."SWITCH_ID_LIGASURE  ", "Source ID"=Control_Fornax_Source_ID."SWITCH_SOURCE_HANDSWITCH  ") -> ("JSON Command"=w437:string)  [unwired: 6 in]
                    n146 = TCP Write(connection ID=w445, data in=w437, 9:100 ("timeout ms (25000)")) -> (connection ID out=w444:refnum<k5>)  [unwired: 1 in, 2 out]
                  }
                }
              }
              frame Default {
                n147 = One Button Dialog(message="This mode is not allowed for this port") -> ()  [unwired: 1 in, 1 out]
              }
            }
          }
        }
      }
      frame "Bipolar Activate Port" {
        n148 = Variant To Data(type=T22 FALSE ("Bipolar Activate"), Variant=w455) -> (data=w454:T22)  [unwired: 1 in, 1 out]
        n149 = call "FT10_Fornax Bipolar Activate Port Command.vi"("Bipolar Activate"=w454, "TCP Network Connection in"=w453) -> ("TCP Network Connection out"=w452:refnum<k5>)  [unwired: 9 in]
      }
      frame "Bipolar Decrease Power" {
        # "Decrease Bipolar Power"
        n150 = call "FT10_Fornax Energy Parameter Command.vi"("Energy Channel ID"=Control_Fornax_Energy_Channel_ID."EC_BIPOLAR  ", "Generator"=T44 "CAMM_EXT_1234321_AJ1428000", "Instrument Type"=Control_Fornax_Instrument_Type."INSTRUMENT_TYPE_BIPOLAR", "Parameter Type"=Control_Fornax_Parameter_Type."POWER_PARAMETER", "Parameter Value"=T19 2, "Energy Mode"=Control_Fornax_Energy_Mode."BIPOLAR_MODE") -> ("JSON Command"=w462:string)  [unwired: 9 in]
        n151 = TCP Write(connection ID=w463, data in=w462, 9:100 ("timeout ms (25000)")) -> (connection ID out=w459:refnum<k5>)  [unwired: 1 in, 2 out]
        n152 = call "Fornax_Read Tester.vi"("TCP Network Connection in"=w459, "Cluster in"=w457) -> ("TCP Network Connection out"=w458:refnum<k5>, "Cluster out"=w456:T42)  [unwired: 8 in]
      }
      frame "Bipolar Increase Power" {
        # "Increase Bipolar Power"
        n153 = call "FT10_Fornax Energy Parameter Command.vi"("Energy Channel ID"=Control_Fornax_Energy_Channel_ID."EC_BIPOLAR  ", "Generator"=T44 "CAMM_EXT_1234321_AJ1428000", "Instrument Type"=Control_Fornax_Instrument_Type."INSTRUMENT_TYPE_BIPOLAR", "Parameter Type"=Control_Fornax_Parameter_Type."POWER_PARAMETER", "Parameter Value"=T19 1, "Energy Mode"=Control_Fornax_Energy_Mode."BIPOLAR_MODE") -> ("JSON Command"=w477:string)  [unwired: 9 in]
        n154 = TCP Write(connection ID=w484, data in=w477, 9:100 ("timeout ms (25000)")) -> (connection ID out=w473:refnum<k5>)  [unwired: 1 in, 2 out]
        n155 = call "Fornax_Read Tester.vi"("TCP Network Connection in"=w473, "Cluster in"=w472) -> ("TCP Network Connection out"=w474:refnum<k5>, "Cluster out"=w471:T42)  [unwired: 8 in]
      }
      frame "Bipolar Mode" {
        n156 = Variant To Data(type=Control_Fornax_Bipolar_Enum."Standard" ("Bipolar Enum"), Variant=w495) -> (data=w493:T23)  [unwired: 1 in, 1 out]
        n157 = call "FT10_Fornax Bipolar Mode Command.vi"("Bipolar Enum in"=w493) -> ("JSON Command"=w490:string)  [unwired: 9 in, 1 out]
        n158 = TCP Write(connection ID=w496, data in=w490, 9:100 ("timeout ms (25000)")) -> (connection ID out=w489:refnum<k5>)  [unwired: 1 in, 2 out]
        n159 = call "Fornax_Read Tester.vi"("TCP Network Connection in"=w489, "Cluster in"=w487) -> ("TCP Network Connection out"=w488:refnum<k5>, "Cluster out"=w486:T42)  [unwired: 8 in]
      }
      frame "Mono1 Cut Activate Port" {
        n160 = Variant To Data(type=T35 FALSE ("Mono1 Cut Activate"), Variant=w505) -> (data=w500:T35)  [unwired: 1 in, 1 out]
        n161 = call "FT10_Fornax Mono1 Cut Activate Port Command.vi"("Mono1 Cut Activate"=w500, "TCP Network Connection in"=w502) -> ("TCP Network Connection out"=w501:refnum<k5>)  [unwired: 9 in]
      }
      frame "Mono1 Cut Decrease Power" {
        # "Decrease Mono1 Cut Power"
        n162 = call "FT10_Fornax Energy Parameter Command.vi"("Energy Channel ID"=Control_Fornax_Energy_Channel_ID."EC_MONO_1  ", "Generator"=T44 "CAMM_EXT_1234321_AJ1428000", "Instrument Type"=Control_Fornax_Instrument_Type."INSTRUMENT_TYPE_MONOPOLAR", "Parameter Type"=Control_Fornax_Parameter_Type."CUT_MODALITY_POWER_PARAMETER", "Parameter Value"=T19 2, "Energy Mode"=Control_Fornax_Energy_Mode."CUT_MODE") -> ("JSON Command"=w510:string)  [unwired: 9 in]
        n163 = TCP Write(connection ID=w519, data in=w510, 9:100 ("timeout ms (25000)")) -> (connection ID out=w509:refnum<k5>)  [unwired: 1 in, 2 out]
        n164 = call "Fornax_Read Tester.vi"("TCP Network Connection in"=w509, "Cluster in"=w507) -> ("TCP Network Connection out"=w508:refnum<k5>, "Cluster out"=w506:T42)  [unwired: 8 in]
      }
      frame "Mono1 Cut Increase Power" {
        # "Increase Mono1 Cut Power"
        n165 = call "FT10_Fornax Energy Parameter Command.vi"("Energy Channel ID"=Control_Fornax_Energy_Channel_ID."EC_MONO_1  ", "Generator"=T44 "CAMM_EXT_1234321_AJ1428000", "Instrument Type"=Control_Fornax_Instrument_Type."INSTRUMENT_TYPE_MONOPOLAR", "Parameter Type"=Control_Fornax_Parameter_Type."CUT_MODALITY_POWER_PARAMETER", "Parameter Value"=T19 1, "Energy Mode"=Control_Fornax_Energy_Mode."CUT_MODE") -> ("JSON Command"=w525:string)  [unwired: 9 in]
        n166 = TCP Write(connection ID=w534, data in=w525, 9:100 ("timeout ms (25000)")) -> (connection ID out=w524:refnum<k5>)  [unwired: 1 in, 2 out]
        n167 = call "Fornax_Read Tester.vi"("TCP Network Connection in"=w524, "Cluster in"=w522) -> ("TCP Network Connection out"=w523:refnum<k5>, "Cluster out"=w521:T42)  [unwired: 8 in]
      }
      frame "Mono1 Cut Mode" {
        n168 = Variant To Data(type=Control_Fornax_Mono1_Cut_Enum."Pure" ("Mono1 Cut Enum"), Variant=w545) -> (data=w542:T37)  [unwired: 1 in, 1 out]
        n169 = call "FT10_Fornax Mono1 Cut Mode Command.vi"("Mono1 Cut Enum in"=w542) -> ("JSON Command"=w540:string)  [unwired: 9 in, 1 out]
        n170 = TCP Write(connection ID=w546, data in=w540, 9:100 ("timeout ms (25000)")) -> (connection ID out=w539:refnum<k5>)  [unwired: 1 in, 2 out]
        n171 = call "Fornax_Read Tester.vi"("TCP Network Connection in"=w539, "Cluster in"=w537) -> ("TCP Network Connection out"=w538:refnum<k5>, "Cluster out"=w536:T42)  [unwired: 8 in]
      }
      frame "Mono1 Coag Activate Port" {
        n172 = Variant To Data(type=T34 FALSE ("Mono1 Coag Activate"), Variant=w555) -> (data=w549:T34)  [unwired: 1 in, 1 out]
        n173 = call "FT10_Fornax Mono1 Coag Activate Port Command.vi"("Mono1 Coag Activate"=w549, "TCP Network Connection in"=w551) -> ("TCP Network Connection out"=w550:refnum<k5>)  [unwired: 9 in]
      }
      frame "Mono1 Coag Decrease Power" {
        # "Decrease Mono1 Coag Power"
        n174 = call "FT10_Fornax Energy Parameter Command.vi"("Energy Channel ID"=Control_Fornax_Energy_Channel_ID."EC_MONO_1  ", "Generator"=T44 "CAMM_EXT_1234321_AJ1428000", "Instrument Type"=Control_Fornax_Instrument_Type."INSTRUMENT_TYPE_MONOPOLAR", "Parameter Type"=Control_Fornax_Parameter_Type."COAG_MODALITY_POWER_PARAMETER", "Parameter Value"=T19 2, "Energy Mode"=Control_Fornax_Energy_Mode."FULGERATE_MODE") -> ("JSON Command"=w560:string)  [unwired: 9 in]
        n175 = TCP Write(connection ID=w569, data in=w560, 9:100 ("timeout ms (25000)")) -> (connection ID out=w559:refnum<k5>)  [unwired: 1 in, 2 out]
        n176 = call "Fornax_Read Tester.vi"("TCP Network Connection in"=w559, "Cluster in"=w557) -> ("TCP Network Connection out"=w558:refnum<k5>, "Cluster out"=w556:T42)  [unwired: 8 in]
      }
      frame "Mono1 Coag Increase Power" {
        # "Increase Mono1 Coag Power"
        n177 = call "FT10_Fornax Energy Parameter Command.vi"("Energy Channel ID"=Control_Fornax_Energy_Channel_ID."EC_MONO_1  ", "Generator"=T44 "CAMM_EXT_1234321_AJ1428000", "Instrument Type"=Control_Fornax_Instrument_Type."INSTRUMENT_TYPE_MONOPOLAR", "Parameter Type"=Control_Fornax_Parameter_Type."COAG_MODALITY_POWER_PARAMETER", "Parameter Value"=T19 1, "Energy Mode"=Control_Fornax_Energy_Mode."FULGERATE_MODE") -> ("JSON Command"=w575:string)  [unwired: 9 in]
        n178 = TCP Write(connection ID=w584, data in=w575, 9:100 ("timeout ms (25000)")) -> (connection ID out=w574:refnum<k5>)  [unwired: 1 in, 2 out]
        n179 = call "Fornax_Read Tester.vi"("TCP Network Connection in"=w574, "Cluster in"=w572) -> ("TCP Network Connection out"=w573:refnum<k5>, "Cluster out"=w571:T42)  [unwired: 8 in]
      }
      frame "Mono1 Coag Mode" {
        n180 = Variant To Data(type=Control_Fornax_Mono1_Coag_Enum."Fulgerate" ("Mono1 Coag Enum"), Variant=w595) -> (data=w592:T36)  [unwired: 1 in, 1 out]
        n181 = call "FT10_Fornax Mono1 Coag Mode Command.vi"("Mono1 Coag Enum in"=w592) -> ("JSON Command"=w590:string)  [unwired: 9 in, 1 out]
        n182 = TCP Write(connection ID=w596, data in=w590, 9:100 ("timeout ms (25000)")) -> (connection ID out=w589:refnum<k5>)  [unwired: 1 in, 2 out]
        n183 = call "Fornax_Read Tester.vi"("TCP Network Connection in"=w589, "Cluster in"=w587) -> ("TCP Network Connection out"=w588:refnum<k5>, "Cluster out"=w586:T42)  [unwired: 8 in]
      }
      frame "Mono2 Cut Activate Port" {
        n184 = Variant To Data(type=T33 FALSE ("Mono2 Cut Activate"), Variant=w605) -> (data=w601:T33)  [unwired: 1 in, 1 out]
        n185 = call "FT10_Fornax Mono2 Cut Activate Port Command.vi"("Mono2 Cut Activate"=w601, "TCP Network Connection in"=w600) -> ("TCP Network Connection out"=w599:refnum<k5>)  [unwired: 9 in]
      }
      frame "Mono2 Cut Decrease Power" {
        # "Decrease Mono2 Cut Power"
        n186 = call "FT10_Fornax Energy Parameter Command.vi"("Energy Channel ID"=Control_Fornax_Energy_Channel_ID."EC_MONO_2  ", "Generator"=T44 "CAMM_EXT_1234321_AJ1428000", "Instrument Type"=Control_Fornax_Instrument_Type."INSTRUMENT_TYPE_MONOPOLAR", "Parameter Type"=Control_Fornax_Parameter_Type."CUT_MODALITY_POWER_PARAMETER", "Parameter Value"=T19 2, "Energy Mode"=Control_Fornax_Energy_Mode."CUT_MODE") -> ("JSON Command"=w610:string)  [unwired: 9 in]
        n187 = TCP Write(connection ID=w619, data in=w610, 9:100 ("timeout ms (25000)")) -> (connection ID out=w609:refnum<k5>)  [unwired: 1 in, 2 out]
        n188 = call "Fornax_Read Tester.vi"("TCP Network Connection in"=w609, "Cluster in"=w607) -> ("TCP Network Connection out"=w608:refnum<k5>, "Cluster out"=w606:T42)  [unwired: 8 in]
      }
      frame "Mono2 Cut Increase Power" {
        # "Increase Mono2 Cut Power"
        n189 = call "FT10_Fornax Energy Parameter Command.vi"("Energy Channel ID"=Control_Fornax_Energy_Channel_ID."EC_MONO_2  ", "Generator"=T44 "CAMM_EXT_1234321_AJ1428000", "Instrument Type"=Control_Fornax_Instrument_Type."INSTRUMENT_TYPE_MONOPOLAR", "Parameter Type"=Control_Fornax_Parameter_Type."CUT_MODALITY_POWER_PARAMETER", "Parameter Value"=T19 1, "Energy Mode"=Control_Fornax_Energy_Mode."CUT_MODE") -> ("JSON Command"=w625:string)  [unwired: 9 in]
        n190 = TCP Write(connection ID=w634, data in=w625, 9:100 ("timeout ms (25000)")) -> (connection ID out=w624:refnum<k5>)  [unwired: 1 in, 2 out]
        n191 = call "Fornax_Read Tester.vi"("TCP Network Connection in"=w624, "Cluster in"=w622) -> ("TCP Network Connection out"=w623:refnum<k5>, "Cluster out"=w621:T42)  [unwired: 8 in]
      }
      frame "Mono2 Cut Mode" {
        n192 = Variant To Data(type=Control_Fornax_Mono2_Cut_Enum."Pure" ("Mono2 Cut Enum"), Variant=w645) -> (data=w641:T29)  [unwired: 1 in, 1 out]
        n193 = call "FT10_Fornax Mono2 Cut Mode Command.vi"("Mono2 Cut Enum in"=w641) -> ("JSON Command"=w640:string)  [unwired: 9 in, 1 out]
        n194 = TCP Write(connection ID=w646, data in=w640, 9:100 ("timeout ms (25000)")) -> (connection ID out=w639:refnum<k5>)  [unwired: 1 in, 2 out]
        n195 = call "Fornax_Read Tester.vi"("TCP Network Connection in"=w639, "Cluster in"=w637) -> ("TCP Network Connection out"=w638:refnum<k5>, "Cluster out"=w636:T42)  [unwired: 8 in]
      }
      frame "Mono2 Coag Activate Port" {
        n196 = Variant To Data(type=T32 FALSE ("Mono2 Coag Activate"), Variant=w655) -> (data=w650:T32)  [unwired: 1 in, 1 out]
        n197 = call "FT10_Fornax Mono2 Coag Activate Port Command.vi"("Mono2 Coag Activate"=w650, "TCP Network Connection in"=w651) -> ("TCP Network Connection out"=w649:refnum<k5>)  [unwired: 9 in]
      }
      frame "Mono2 Coag Decrease Power" {
        # "Decrease Mono2 Coag Power"
        n198 = call "FT10_Fornax Energy Parameter Command.vi"("Energy Channel ID"=Control_Fornax_Energy_Channel_ID."EC_MONO_2  ", "Generator"=T44 "CAMM_EXT_1234321_AJ1428000", "Instrument Type"=Control_Fornax_Instrument_Type."INSTRUMENT_TYPE_MONOPOLAR", "Parameter Type"=Control_Fornax_Parameter_Type."COAG_MODALITY_POWER_PARAMETER", "Parameter Value"=T19 2, "Energy Mode"=Control_Fornax_Energy_Mode."FULGERATE_MODE") -> ("JSON Command"=w660:string)  [unwired: 9 in]
        n199 = TCP Write(connection ID=w669, data in=w660, 9:100 ("timeout ms (25000)")) -> (connection ID out=w659:refnum<k5>)  [unwired: 1 in, 2 out]
        n200 = call "Fornax_Read Tester.vi"("TCP Network Connection in"=w659, "Cluster in"=w657) -> ("TCP Network Connection out"=w658:refnum<k5>, "Cluster out"=w656:T42)  [unwired: 8 in]
      }
      frame "Mono2 Coag Increase Power" {
        # "Increase Mono2 Coag Power"
        n201 = call "FT10_Fornax Energy Parameter Command.vi"("Energy Channel ID"=Control_Fornax_Energy_Channel_ID."EC_MONO_2  ", "Generator"=T44 "CAMM_EXT_1234321_AJ1428000", "Instrument Type"=Control_Fornax_Instrument_Type."INSTRUMENT_TYPE_MONOPOLAR", "Parameter Type"=Control_Fornax_Parameter_Type."COAG_MODALITY_POWER_PARAMETER", "Parameter Value"=T19 1, "Energy Mode"=Control_Fornax_Energy_Mode."FULGERATE_MODE") -> ("JSON Command"=w675:string)  [unwired: 9 in]
        n202 = TCP Write(connection ID=w684, data in=w675, 9:100 ("timeout ms (25000)")) -> (connection ID out=w674:refnum<k5>)  [unwired: 1 in, 2 out]
        n203 = call "Fornax_Read Tester.vi"("TCP Network Connection in"=w674, "Cluster in"=w672) -> ("TCP Network Connection out"=w673:refnum<k5>, "Cluster out"=w671:T42)  [unwired: 8 in]
      }
      frame "Mono2 Coag Mode" {
        n204 = Variant To Data(type=Control_Fornax_Mono2_Coag_Enum."Fulgerate" ("Mono2 Coag Enum"), Variant=w695) -> (data=w692:T26)  [unwired: 1 in, 1 out]
        n205 = call "FT10_Fornax Mono2 Coag Mode Command.vi"("Mono2 Coag Enum in"=w692) -> ("JSON Command"=w690:string)  [unwired: 9 in, 1 out]
        n206 = TCP Write(connection ID=w696, data in=w690, 9:100 ("timeout ms (25000)")) -> (connection ID out=w689:refnum<k5>)  [unwired: 1 in, 2 out]
        n207 = call "Fornax_Read Tester.vi"("TCP Network Connection in"=w689, "Cluster in"=w687) -> ("TCP Network Connection out"=w688:refnum<k5>, "Cluster out"=w686:T42)  [unwired: 8 in]
      }
      frame "Ligasure Activate Port" {
        n208 = Variant To Data(type=T21 FALSE ("Ligasure Activate"), Variant=w705) -> (data=w701:T21)  [unwired: 1 in, 1 out]
        n209 = call "FT10_Fornax Ligasure Activate Port Command.vi"("Ligasure Activate"=w701, "TCP Network Connection in"=w702) -> ("TCP Network Connection out"=w700:refnum<k5>)  [unwired: 9 in]
      }
      frame "Exit" {
        n210 = local write "Display Message"("\"Stop\" button pressed" ("Display Message")) -> ()
      }
    }
  }
  n211 = while {
    tunnel: w20 -> [w714]
    shift-right: [w712] -> _
    shift-left: _ -> [w711]
    stop <- w713 stop-if-true
    n212 = event shown="[21] \"Mono1 Cut plus\": Value Change" {
      selector: _ -> [_ _ _ _ _ _ _ _ _ _ _ _ _ _ _ _ _ _ _ _ _ _ _ _ _ _ _ _ _ _ _ _ _ _ _ _ _]
      dyn-events: _ -> [_ _ _ _ _ _ _ _ _ _ _ _ _ _ _ _ _ _ _ _ _ _ _ _ _ _ _ _ _ _ _ _ _ _ _ _ _]
      timeout: _ -> [_ _ _ _ _ _ _ _ _ _ _ _ _ _ _ _ _ _ _ _ _ _ _ _ _ _ _ _ _ _ _ _ _ _ _ _ _]
      tunnel: w714 -> [w717 w721 w725 w729 w733 w737 w741 w745 w751 w757 w763 w769 w775 _ w791 w802 w811 w818 w825 w833 w842 w849 w856 w864 w873 w880 w887 w895 w904 w911 w918 w926 w935 w942 w949 w957 w965]
      tunnel: [FALSE FALSE FALSE FALSE FALSE FALSE FALSE FALSE FALSE FALSE FALSE FALSE FALSE FALSE FALSE FALSE FALSE FALSE FALSE FALSE FALSE FALSE FALSE FALSE FALSE FALSE FALSE FALSE FALSE FALSE FALSE FALSE FALSE FALSE FALSE FALSE TRUE] -> w713
      tunnel: [w715 w719 w723 w727 w731 w735 w739 w743 w747 w753 w759 w765 w771 w778 w789 w799 w809 w816 w822 w830 w840 w847 w854 w861 w871 w878 w885 w892 w902 w909 w916 w923 w933 w940 w947 w954 w963] -> w712
      tunnel: w711 -> [w715 w719 w723 w727 w731 w735 w739 w743 w747 w753 w759 w765 w771 _ w789 w799 w809 w816 w822 w830 w840 w847 w854 w861 w871 w878 w885 w892 w902 w909 w916 w923 w933 w940 w947 w954 w963]
      event "Action 1": Value Change {
        n213 = event-data() -> ()  [unwired: 1 in, 4 out]
        n214 = Enqueue Element(queue=w717, element=T43 {"Message"="Fornax Action 1", "Message Data"=variant}) -> ()  [unwired: 2 in, 3 out]
      }
      event "Set Monopolar Command": Value Change {
        n215 = event-data() -> ()  [unwired: 1 in, 2 out]
        n216 = Enqueue Element(queue=w721, element=T43 {"Message"="Fornax Set Monopolar Command", "Message Data"=variant}) -> ()  [unwired: 2 in, 3 out]
      }
      event "Send String Array Command": Value Change {
        n217 = event-data() -> ()  [unwired: 1 in, 3 out]
        n218 = Enqueue Element(queue=w725, element=T43 {"Message"="Send String Array Command", "Message Data"=variant}) -> ()  [unwired: 2 in, 3 out]
      }
      event "Send String Command": Value Change {
        n219 = event-data() -> ()  [unwired: 1 in, 2 out]
        n220 = Enqueue Element(queue=w729, element=T43 {"Message"="Send String Command", "Message Data"=variant}) -> ()  [unwired: 2 in, 3 out]
      }
      event "Send Read Command": Value Change {
        n221 = event-data() -> ()  [unwired: 1 in, 4 out]
        n222 = Enqueue Element(queue=w733, element=T43 {"Message"="Send Read Command", "Message Data"=variant}) -> ()  [unwired: 2 in, 3 out]
      }
      event "Other Read Command": Value Change {
        n223 = event-data() -> ()  [unwired: 1 in, 4 out]
        n224 = Enqueue Element(queue=w737, element=T43 {"Message"="Other Read Command", "Message Data"=variant}) -> ()  [unwired: 2 in, 3 out]
      }
      event "Slow Read": Value Change {
        n225 = event-data() -> ()  [unwired: 1 in, 4 out]
        n226 = Enqueue Element(queue=w741, element=T43 {"Message"="Slow Read", "Message Data"=variant}) -> ()  [unwired: 2 in, 3 out]
      }
      event "Test Read": Value Change {
        n227 = event-data() -> ()  [unwired: 1 in, 4 out]
        n228 = Enqueue Element(queue=w745, element=T43 {"Message"="Test Read", "Message Data"=variant}) -> ()  [unwired: 2 in, 3 out]
      }
      event "External Command": Value Change {
        n229 = event-data() -> ()  [unwired: 1 in, 4 out]
        n230 = Bundle By Name(cluster=T43 {"Message"="", "Message Data"=variant} ("element"), "Message"="External Command") -> (w749:T43)
        n231 = Enqueue Element(queue=w751, element=w749) -> ()  [unwired: 2 in, 3 out]
      }
      event "System Config": Value Change {
        n232 = event-data() -> ()  [unwired: 1 in, 3 out]
        n233 = Bundle By Name(cluster=T43 {"Message"="", "Message Data"=variant} ("element"), "Message"="System Config") -> (w755:T43)
        n234 = Enqueue Element(queue=w757, element=w755) -> ()  [unwired: 2 in, 3 out]
      }
      event "Switch Status Command": Value Change {
        n235 = event-data() -> ()  [unwired: 1 in, 3 out]
        n236 = Bundle By Name(cluster=T43 {"Message"="", "Message Data"=variant} ("element"), "Message"="Switch Status Command") -> (w761:T43)
        n237 = Enqueue Element(queue=w763, element=w761) -> ()  [unwired: 2 in, 3 out]
      }
      event "Slider Status Command": Value Change {
        n238 = event-data() -> ()  [unwired: 1 in, 2 out]
        n239 = Bundle By Name(cluster=T43 {"Message"="", "Message Data"=variant} ("element"), "Message"="Slider Status Command") -> (w767:T43)
        n240 = Enqueue Element(queue=w769, element=w767) -> ()  [unwired: 2 in, 3 out]
      }
      event "Energy Parameter Command": Value Change {
        n241 = event-data() -> ()  [unwired: 1 in, 1 out]
        n242 = Bundle By Name(cluster=T43 {"Message"="", "Message Data"=variant} ("element"), "Message"="Energy Parameter Command") -> (w773:T43)
        n243 = Enqueue Element(queue=w775, element=w773) -> ()  [unwired: 2 in, 3 out]
      }
      event "Port": Value Change {
        n244 = event-data() -> ()  [unwired: 1 in, 1 out]
        n245 = case shown="\"Ligasure\"" "Port" {
          selector: "Port" -> [w780 w782 w784 w786]
          tunnel: [w780 w782 w784 w786] -> w778
          frame "Mono1", Default {
            # "Modes:\n0 - Cut\n1 - Coag\n2 - Bipolar\n3 - Ligasure"
            n246 = property on="Mode" class="Enum (strict)"("Disabled Items []"=i32[] [2, 3]) -> ()  [unwired: 2 in, 2 out]
          }
          frame "Mono2" {
            # "Modes:\n0 - Cut\n1 - Coag\n2 - Bipolar\n3 - Ligasure"
            n247 = property on="Mode" class="Enum (strict)"("Disabled Items []"=i32[] [2, 3]) -> ()  [unwired: 2 in, 2 out]
          }
          frame "Bipolar" {
            # "Modes:\n0 - Cut\n1 - Coag\n2 - Bipolar\n3 - Ligasure"
            n248 = property on="Mode" class="Enum (strict)"("Disabled Items []"=i32[] [0, 1, 3]) -> ()  [unwired: 2 in, 2 out]
          }
          frame "Ligasure" {
            # "Modes:\n0 - Cut\n1 - Coag\n2 - Bipolar\n3 - Ligasure"
            n249 = property on="Mode" class="Enum (strict)"("Disabled Items []"=i32[] [0, 1, 2]) -> ()  [unwired: 2 in, 2 out]
          }
        }
      }
      event "On/Off": Value Change {
        n250 = event-data() -> ()  [unwired: 1 in, 1 out]
        n251 = Bundle By Name(cluster=T45 {"Port"=enum."Bipolar", "Mode"=enum."Bipolar", "On/Off"=FALSE}, "Port"=w789, "Mode"="Mode", "On/Off"="On/Off") -> (w790:T45)
        n252 = Bundle By Name(cluster=T43 {"Message"="", "Message Data"=variant} ("element"), "Message Data"=w790, "Message"="Activate Port") -> (w793:T43)
        n253 = Enqueue Element(queue=w791, element=w793) -> ()  [unwired: 2 in, 3 out]
      }
      event Value Change {
        n254 = event-data() -> ()  [unwired: 1 in, 1 out]
        n255 = case shown="True" "Bipolar Activate" {
          tunnel: ["Deactivate" ("Message") "Activate" ("Message")] -> w801
          frame True {
          }
          frame False {
          }
        }
        n256 = property on="Bipolar Activate" class="Bool (strict)"("BoolText.Text"=w801) -> ()  [unwired: 2 in, 2 out]
        n257 = Bundle By Name(cluster=T43 {"Message"="", "Message Data"=variant} ("element"), "Message Data"="Bipolar Activate", "Message"="Bipolar Activate Port") -> (w804:T43)
        n258 = Enqueue Element(queue=w802, element=w804) -> ()  [unwired: 2 in, 3 out]
      }
      event Value Change {
        n259 = event-data() -> ()  [unwired: 1 in, 1 out]
        n260 = Bundle By Name(cluster=T43 {"Message"="", "Message Data"=variant} ("element"), "Message Data"="Bipolar minus", "Message"="Bipolar Decrease Power") -> (w813:T43)
        n261 = Enqueue Element(queue=w811, element=w813) -> ()  [unwired: 2 in, 3 out]
      }
      event Value Change {
        n262 = event-data() -> ()  [unwired: 1 in, 1 out]
        n263 = Bundle By Name(cluster=T43 {"Message"="", "Message Data"=variant} ("element"), "Message Data"="Bipolar plus", "Message"="Bipolar Increase Power") -> (w820:T43)
        n264 = Enqueue Element(queue=w818, element=w820) -> ()  [unwired: 2 in, 3 out]
      }
      event Value Change {
        n265 = event-data() -> ()  [unwired: 1 in, 1 out]
        n266 = Bundle By Name(cluster=T43 {"Message"="", "Message Data"=variant} ("element"), "Message Data"="Bipolar Enum", "Message"="Bipolar Mode") -> (w827:T43)
        n267 = Enqueue Element(queue=w825, element=w827) -> ()  [unwired: 2 in, 3 out]
      }
      event Value Change {
        n268 = event-data() -> ()  [unwired: 1 in, 4 out]
        n269 = case shown="True" "Mono1 Cut Activate" {
          tunnel: ["Deactivate" ("Message") "Activate" ("Message")] -> w832
          frame True {
          }
          frame False {
          }
        }
        n270 = property on="Mono1 Cut Activate" class="Bool (strict)"("BoolText.Text"=w832) -> ()  [unwired: 2 in, 2 out]
        n271 = Bundle By Name(cluster=T43 {"Message"="", "Message Data"=variant} ("element"), "Message Data"="Mono1 Cut Activate", "Message"="Mono1 Cut Activate Port") -> (w835:T43)
        n272 = Enqueue Element(queue=w833, element=w835) -> ()  [unwired: 2 in, 3 out]
      }
      event Value Change {
        n273 = event-data() -> ()  [unwired: 1 in, 4 out]
        n274 = Bundle By Name(cluster=T43 {"Message"="", "Message Data"=variant} ("element"), "Message Data"="Mono1 Cut minus", "Message"="Mono1 Cut Decrease Power") -> (w844:T43)
        n275 = Enqueue Element(queue=w842, element=w844) -> ()  [unwired: 2 in, 3 out]
      }
      event Value Change {
        n276 = event-data() -> ()  [unwired: 1 in, 4 out]
        n277 = Bundle By Name(cluster=T43 {"Message"="", "Message Data"=variant} ("element"), "Message Data"="Mono1 Cut plus", "Message"="Mono1 Cut Increase Power") -> (w851:T43)
        n278 = Enqueue Element(queue=w849, element=w851) -> ()  [unwired: 2 in, 3 out]
      }
      event Value Change {
        n279 = event-data() -> ()  [unwired: 1 in, 4 out]
        n280 = Bundle By Name(cluster=T43 {"Message"="", "Message Data"=variant} ("element"), "Message Data"="Mono1 Cut Enum", "Message"="Mono1 Cut Mode") -> (w858:T43)
        n281 = Enqueue Element(queue=w856, element=w858) -> ()  [unwired: 2 in, 3 out]
      }
      event Value Change {
        n282 = event-data() -> ()  [unwired: 1 in, 4 out]
        n283 = case shown="True" "Mono1 Coag Activate" {
          tunnel: ["Deactivate" ("Message") "Activate" ("Message")] -> w862
          frame True {
          }
          frame False {
          }
        }
        n284 = property on="Mono1 Coag Activate" class="Bool (strict)"("BoolText.Text"=w862) -> ()  [unwired: 2 in, 2 out]
        n285 = Bundle By Name(cluster=T43 {"Message"="", "Message Data"=variant} ("element"), "Message Data"="Mono1 Coag Activate", "Message"="Mono1 Coag Activate Port") -> (w866:T43)
        n286 = Enqueue Element(queue=w864, element=w866) -> ()  [unwired: 2 in, 3 out]
      }
      event Value Change {
        n287 = event-data() -> ()  [unwired: 1 in, 4 out]
        n288 = Bundle By Name(cluster=T43 {"Message"="", "Message Data"=variant} ("element"), "Message Data"="Mono1 Coag minus", "Message"="Mono1 Coag Decrease Power") -> (w875:T43)
        n289 = Enqueue Element(queue=w873, element=w875) -> ()  [unwired: 2 in, 3 out]
      }
      event Value Change {
        n290 = event-data() -> ()  [unwired: 1 in, 4 out]
        n291 = Bundle By Name(cluster=T43 {"Message"="", "Message Data"=variant} ("element"), "Message Data"="Mono1 Coag plus", "Message"="Mono1 Coag Increase Power") -> (w882:T43)
        n292 = Enqueue Element(queue=w880, element=w882) -> ()  [unwired: 2 in, 3 out]
      }
      event Value Change {
        n293 = event-data() -> ()  [unwired: 1 in, 4 out]
        n294 = Bundle By Name(cluster=T43 {"Message"="", "Message Data"=variant} ("element"), "Message Data"="Mono1 Coag Enum", "Message"="Mono1 Coag Mode") -> (w889:T43)
        n295 = Enqueue Element(queue=w887, element=w889) -> ()  [unwired: 2 in, 3 out]
      }
      event Value Change {
        n296 = event-data() -> ()  [unwired: 1 in, 4 out]
        n297 = case shown="True" "Mono2 Cut Activate" {
          tunnel: ["Deactivate" ("Message") "Activate" ("Message")] -> w894
          frame True {
          }
          frame False {
          }
        }
        n298 = property on="Mono2 Cut Activate" class="Bool (strict)"("BoolText.Text"=w894) -> ()  [unwired: 2 in, 2 out]
        n299 = Bundle By Name(cluster=T43 {"Message"="", "Message Data"=variant} ("element"), "Message Data"="Mono2 Cut Activate", "Message"="Mono2 Cut Activate Port") -> (w897:T43)
        n300 = Enqueue Element(queue=w895, element=w897) -> ()  [unwired: 2 in, 3 out]
      }
      event Value Change {
        n301 = event-data() -> ()  [unwired: 1 in, 4 out]
        n302 = Bundle By Name(cluster=T43 {"Message"="", "Message Data"=variant} ("element"), "Message Data"="Mono2 Cut minus", "Message"="Mono2 Cut Decrease Power") -> (w906:T43)
        n303 = Enqueue Element(queue=w904, element=w906) -> ()  [unwired: 2 in, 3 out]
      }
      event Value Change {
        n304 = event-data() -> ()  [unwired: 1 in, 4 out]
        n305 = Bundle By Name(cluster=T43 {"Message"="", "Message Data"=variant} ("element"), "Message Data"="Mono2 Cut plus", "Message"="Mono2 Cut Increase Power") -> (w913:T43)
        n306 = Enqueue Element(queue=w911, element=w913) -> ()  [unwired: 2 in, 3 out]
      }
      event Value Change {
        n307 = event-data() -> ()  [unwired: 1 in, 4 out]
        n308 = Bundle By Name(cluster=T43 {"Message"="", "Message Data"=variant} ("element"), "Message Data"="Mono2 Cut Enum", "Message"="Mono2 Cut Mode") -> (w920:T43)
        n309 = Enqueue Element(queue=w918, element=w920) -> ()  [unwired: 2 in, 3 out]
      }
      event Value Change {
        n310 = event-data() -> ()  [unwired: 1 in, 4 out]
        n311 = case shown="True" "Mono2 Coag Activate" {
          tunnel: ["Deactivate" ("Message") "Activate" ("Message")] -> w925
          frame True {
          }
          frame False {
          }
        }
        n312 = property on="Mono2 Coag Activate" class="Bool (strict)"("BoolText.Text"=w925) -> ()  [unwired: 2 in, 2 out]
        n313 = Bundle By Name(cluster=T43 {"Message"="", "Message Data"=variant} ("element"), "Message Data"="Mono2 Coag Activate", "Message"="Mono2 Coag Activate Port") -> (w928:T43)
        n314 = Enqueue Element(queue=w926, element=w928) -> ()  [unwired: 2 in, 3 out]
      }
      event Value Change {
        n315 = event-data() -> ()  [unwired: 1 in, 4 out]
        n316 = Bundle By Name(cluster=T43 {"Message"="", "Message Data"=variant} ("element"), "Message Data"="Mono2 Coag minus", "Message"="Mono2 Coag Decrease Power") -> (w937:T43)
        n317 = Enqueue Element(queue=w935, element=w937) -> ()  [unwired: 2 in, 3 out]
      }
      event Value Change {
        n318 = event-data() -> ()  [unwired: 1 in, 4 out]
        n319 = Bundle By Name(cluster=T43 {"Message"="", "Message Data"=variant} ("element"), "Message Data"="Mono2 Coag plus", "Message"="Mono2 Coag Increase Power") -> (w944:T43)
        n320 = Enqueue Element(queue=w942, element=w944) -> ()  [unwired: 2 in, 3 out]
      }
      event Value Change {
        n321 = event-data() -> ()  [unwired: 1 in, 4 out]
        n322 = Bundle By Name(cluster=T43 {"Message"="", "Message Data"=variant} ("element"), "Message Data"="Mono2 Coag Enum", "Message"="Mono2 Coag Mode") -> (w951:T43)
        n323 = Enqueue Element(queue=w949, element=w951) -> ()  [unwired: 2 in, 3 out]
      }
      event Value Change {
        n324 = event-data() -> ()  [unwired: 1 in, 4 out]
        n325 = case shown="True" "Ligasure Activate" {
          tunnel: ["Deactivate" ("Message") "Activate" ("Message")] -> w955
          frame True {
          }
          frame False {
          }
        }
        n326 = property on="Ligasure Activate" class="Bool (strict)"("BoolText.Text"=w955) -> ()  [unwired: 2 in, 2 out]
        n327 = Bundle By Name(cluster=T43 {"Message"="", "Message Data"=variant} ("element"), "Message Data"="Ligasure Activate", "Message"="Ligasure Activate Port") -> (w959:T43)
        n328 = Enqueue Element(queue=w957, element=w959) -> ()  [unwired: 2 in, 3 out]
      }
      event "Stop": Value Change {
        n329 = event-data() -> ()  [unwired: 1 in, 5 out]
        n330 = Enqueue Element At Opposite End(queue=w965, element=T43 {"Message"="Exit", "Message Data"=variant}) -> ()  [unwired: 2 in, 3 out]
      }
    }
  }
